vi "MGCC_FntStaMach_Visualization_OpalRT_demo_EvanEdit.vi"() -> ()   [LabVIEW 2016]
uses:
  Communication (Yiwei)/Global communication output.vi
panel:
  in  "test com":dbl[](array[numeric])
  in  "Matrix output":bool
  out "G14":bool
  out "G1":bool
  out "G6":bool
  out "L10":dbl
  in  "Tab Control 4":enum32{"Page 1"}(tab)
  out "PV Forecast":dbl[](graph)
  in  "Tab Control 3":enum32{"Page 1"}(tab)
  out "Sources Power":T1(graph)
  in  "Tab Control 2":enum32{"Page 1"}(tab)
  out "Frequency":T2(graph)
  in  "Irradiance":string(combo)="Manually Control"
  in  "island cmd 2":bool
  out "L11":dbl format="%#_4f"
  out "L9":dbl format="%#_4f"
  out "L7":dbl format="%#_4f"
  out "L8":dbl format="%#_4f"
  out "L4":dbl format="%#_4f"
  out "L3":dbl format="%#.1f"
  out "L2":dbl format="%#_4f"
  out "L5":dbl format="%#_4f"
  out "Total Load":dbl format="%#.1f"
  out "Max PV":dbl format="%#.1f"
  out "Resynchronization":bool
  out "Angle Diff.\n01-02":dbl format="%#.1f"
  out "Angle Diff.\n04-05":dbl format="%#.1f"
  out "Angle Diff.\n03-04":dbl format="%#.1f"
  out "Angle Diff.\n03-07":dbl format="%#.1f"
  out "Angle Diff.\n07-09":dbl format="%#.1f"
  out "Angle Diff.\n10-11":dbl format="%#.1f"
  out "L3":bool
  out "L2":bool
  out "2":cluster{dbl[], dbl[]}(graph)
  out "5":cluster{dbl[], dbl[]}(graph)
  out "4":cluster{dbl[], dbl[]}(graph)
  out "8":cluster{dbl[], dbl[]}(graph)
  out "9":cluster{dbl[], dbl[]}(graph)
  out "11":cluster{dbl[], dbl[]}(graph)
  in  "Stop":bool
  in  "RESET":bool
  out "3":cluster{dbl[], dbl[]}(graph)
  out "7":cluster{dbl[], dbl[]}(graph)
  out "10":cluster{dbl[], dbl[]}(graph)
  out "13":cluster{dbl[], dbl[]}(graph)
  out "14":cluster{dbl[], dbl[]}(graph)
  out "6":cluster{dbl[], dbl[]}(graph)
  out "1":cluster{dbl[], dbl[]}(graph)
  in  "Tab Control":T3(tab)
  out "Node Voltage":dbl(graph)
  out "Node Voltage":dbl(graph)
  out "Node Voltage":dbl(graph)
  out "Node Voltage":dbl(graph)
  out "Node Voltage":dbl(graph)
  out "Node Voltage":dbl(graph)
  out "Node Voltage":dbl(graph)
  out "Node Voltage":dbl(graph)
  out "Node Voltage":dbl(graph)
  out "Reactive power control":bool
  out "Active power control":bool
  out "Communication":bool
  out "Reactive power control":bool
  out "Active power control":bool
  out "Resynchronization":bool
  out "Communication":bool
  in  "Island 3":bool
  in  "Island 2":bool
  in  "Island":bool
  in  "Ready for STD":bool
  in  "Recon cmd":bool
  in  "BKS cmd":bool
  in  "island cmd":bool
  out "Angle Diff.\n11-14":dbl format="%#.1f"
  out "Angle Diff.\n09-10":dbl format="%#.1f"
  out "Angle Diff.\n04-06":dbl format="%#.1f"
  out "Angle Diff.\n 02-03":dbl format="%#.1f"
  out "BESS LC":bool
  out "PV LC":bool
  out "Topology Identification":bool
  out "PV Forecasting":bool
  out "Load Forecasting":bool
  out "PQ Balance":bool
  out "Black Start":bool
  out "Data Logging":bool
  out "Communication":bool
  out "State Estimation":bool
  out "Energy Mgmt.":bool
  out "SOC Tank":dbl(slide) scale=0.0..100.0
  out "S1114":bool
  out "S1011":bool
  out "S1012":bool
  out "S1013":bool
  out "S0910":bool
  out "S0708":bool
  out "S0709":bool
  out "S0307":bool
  out "S0304":bool
  out "S0406":bool
  out "S0405":bool
  out "S0203":bool
  out "S0102":bool
  out "W11":bool
  out "W8":bool
  out "L11":bool
  out "W12":bool
  out "L10":bool
  out "L7":bool
  out "L9":bool
  out "W7":bool
  out "L8":bool
  out "L4":bool
  out "L5":bool
  out "W6":bool
  out "W3":bool
  out "W2":bool
  out "Battery Output":dbl format="%#.1f"
  out "Battery SOC":dbl format="%#.1f"
  in  "PV-12":dbl(slide) scale=0.0..2.0
  out "PV Output":dbl format="%#.1f"
  out "W4":bool
  out "Current State":string
  out "W9":bool
  # "A Smart and Flexible Microgrid with a Low-cost Scalable Open-source Controller"
  # "Microgrid Central Controller"
  # "Battery Local Controller"
  # "%"
  # "G-6"
  # "kW"
  # "kW"
  # "kW"
  # "kW"
  # "kW"
  # "G-14"
  # "kW"
  # "kW"
  # "Deg"
  # "kW"
  # "Deg"
  # "Deg"
  # "kW"
  # "G-1"
  # "Deg"
  # "Deg"
  # "Deg"
  # "Deg"
  # "kW"
  # "Deg"
  # "kW"
  # "PV Local Controller"
  # "Deg"
  # "kW"
  # "kW"
  # "Deg"
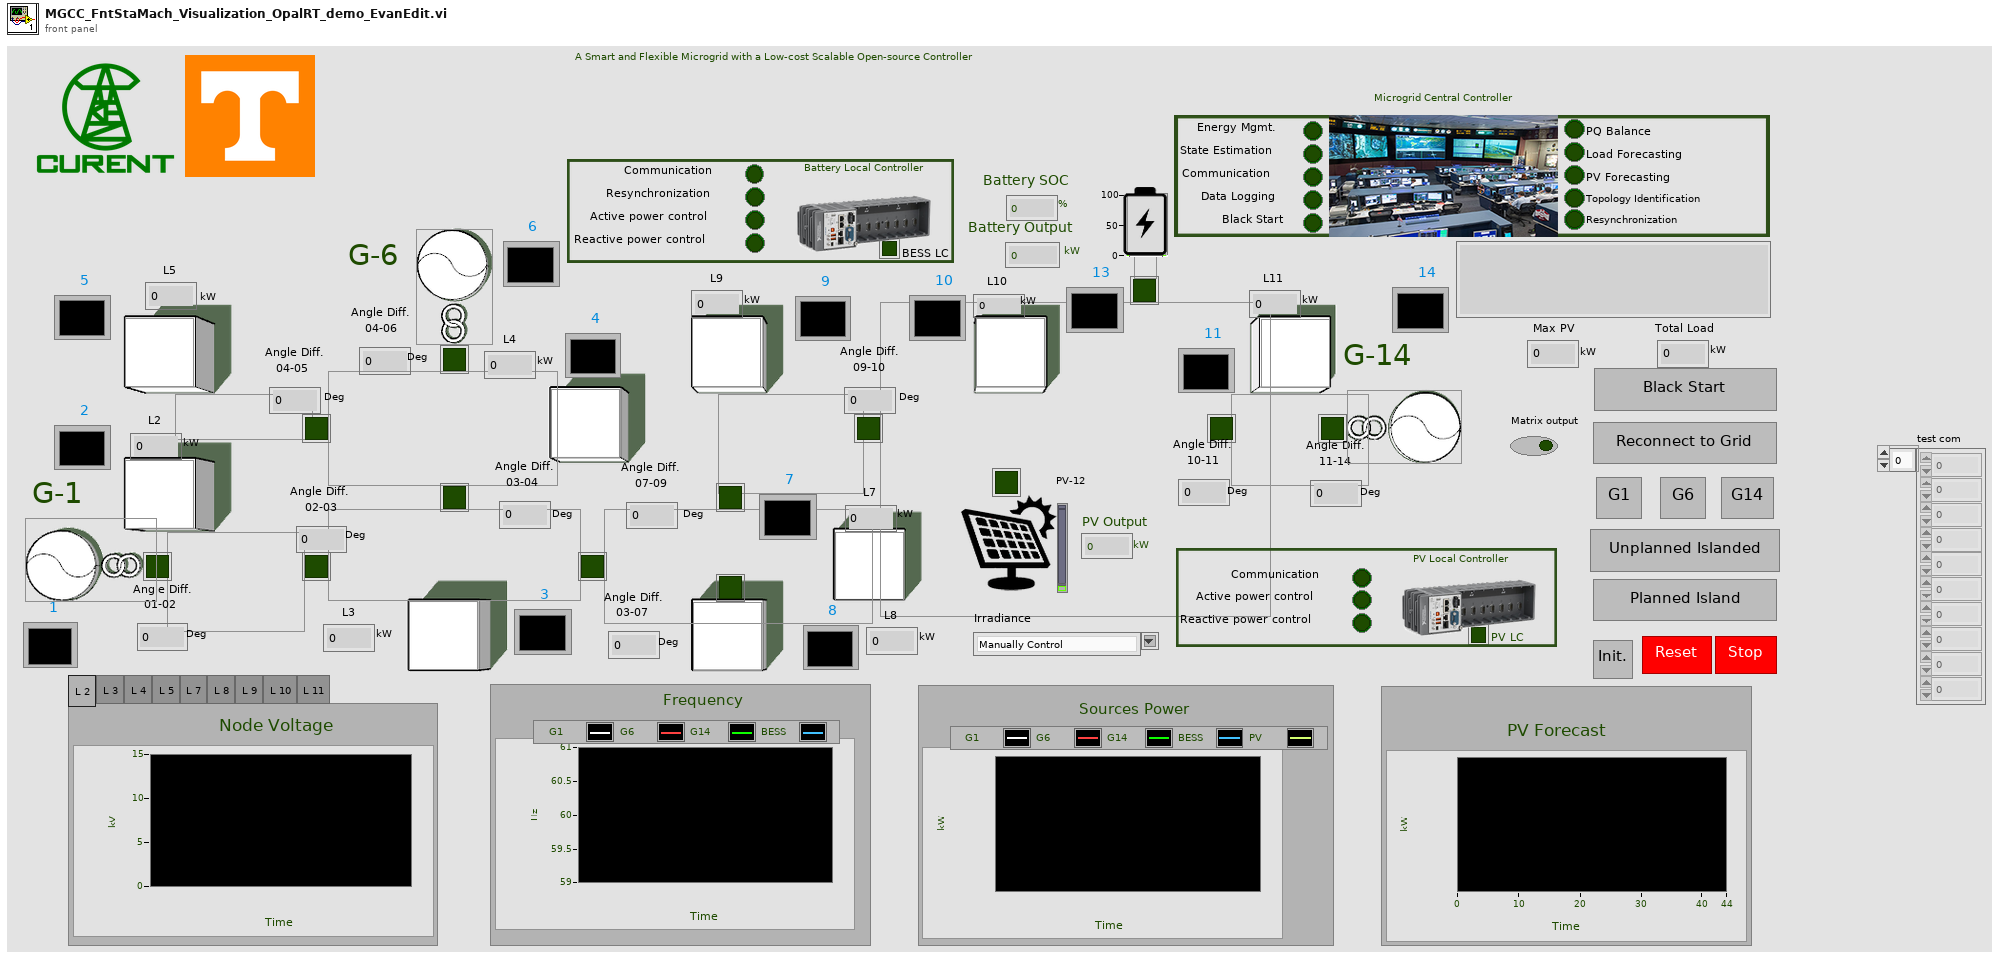
[diagram p1: front panel]
types:
  T1 = cluster{"Double":dbl, "Double":dbl, "Double":dbl, "Double":dbl, "Double":dbl}
  T2 = cluster{"Double":dbl, "Double":dbl, "Double":dbl, "Double":dbl}
  T3 = enum32{"L 2", "L 3", "L 4", "L 5", "L 7", "L 8", "L 9", "L 10", "L 11"}
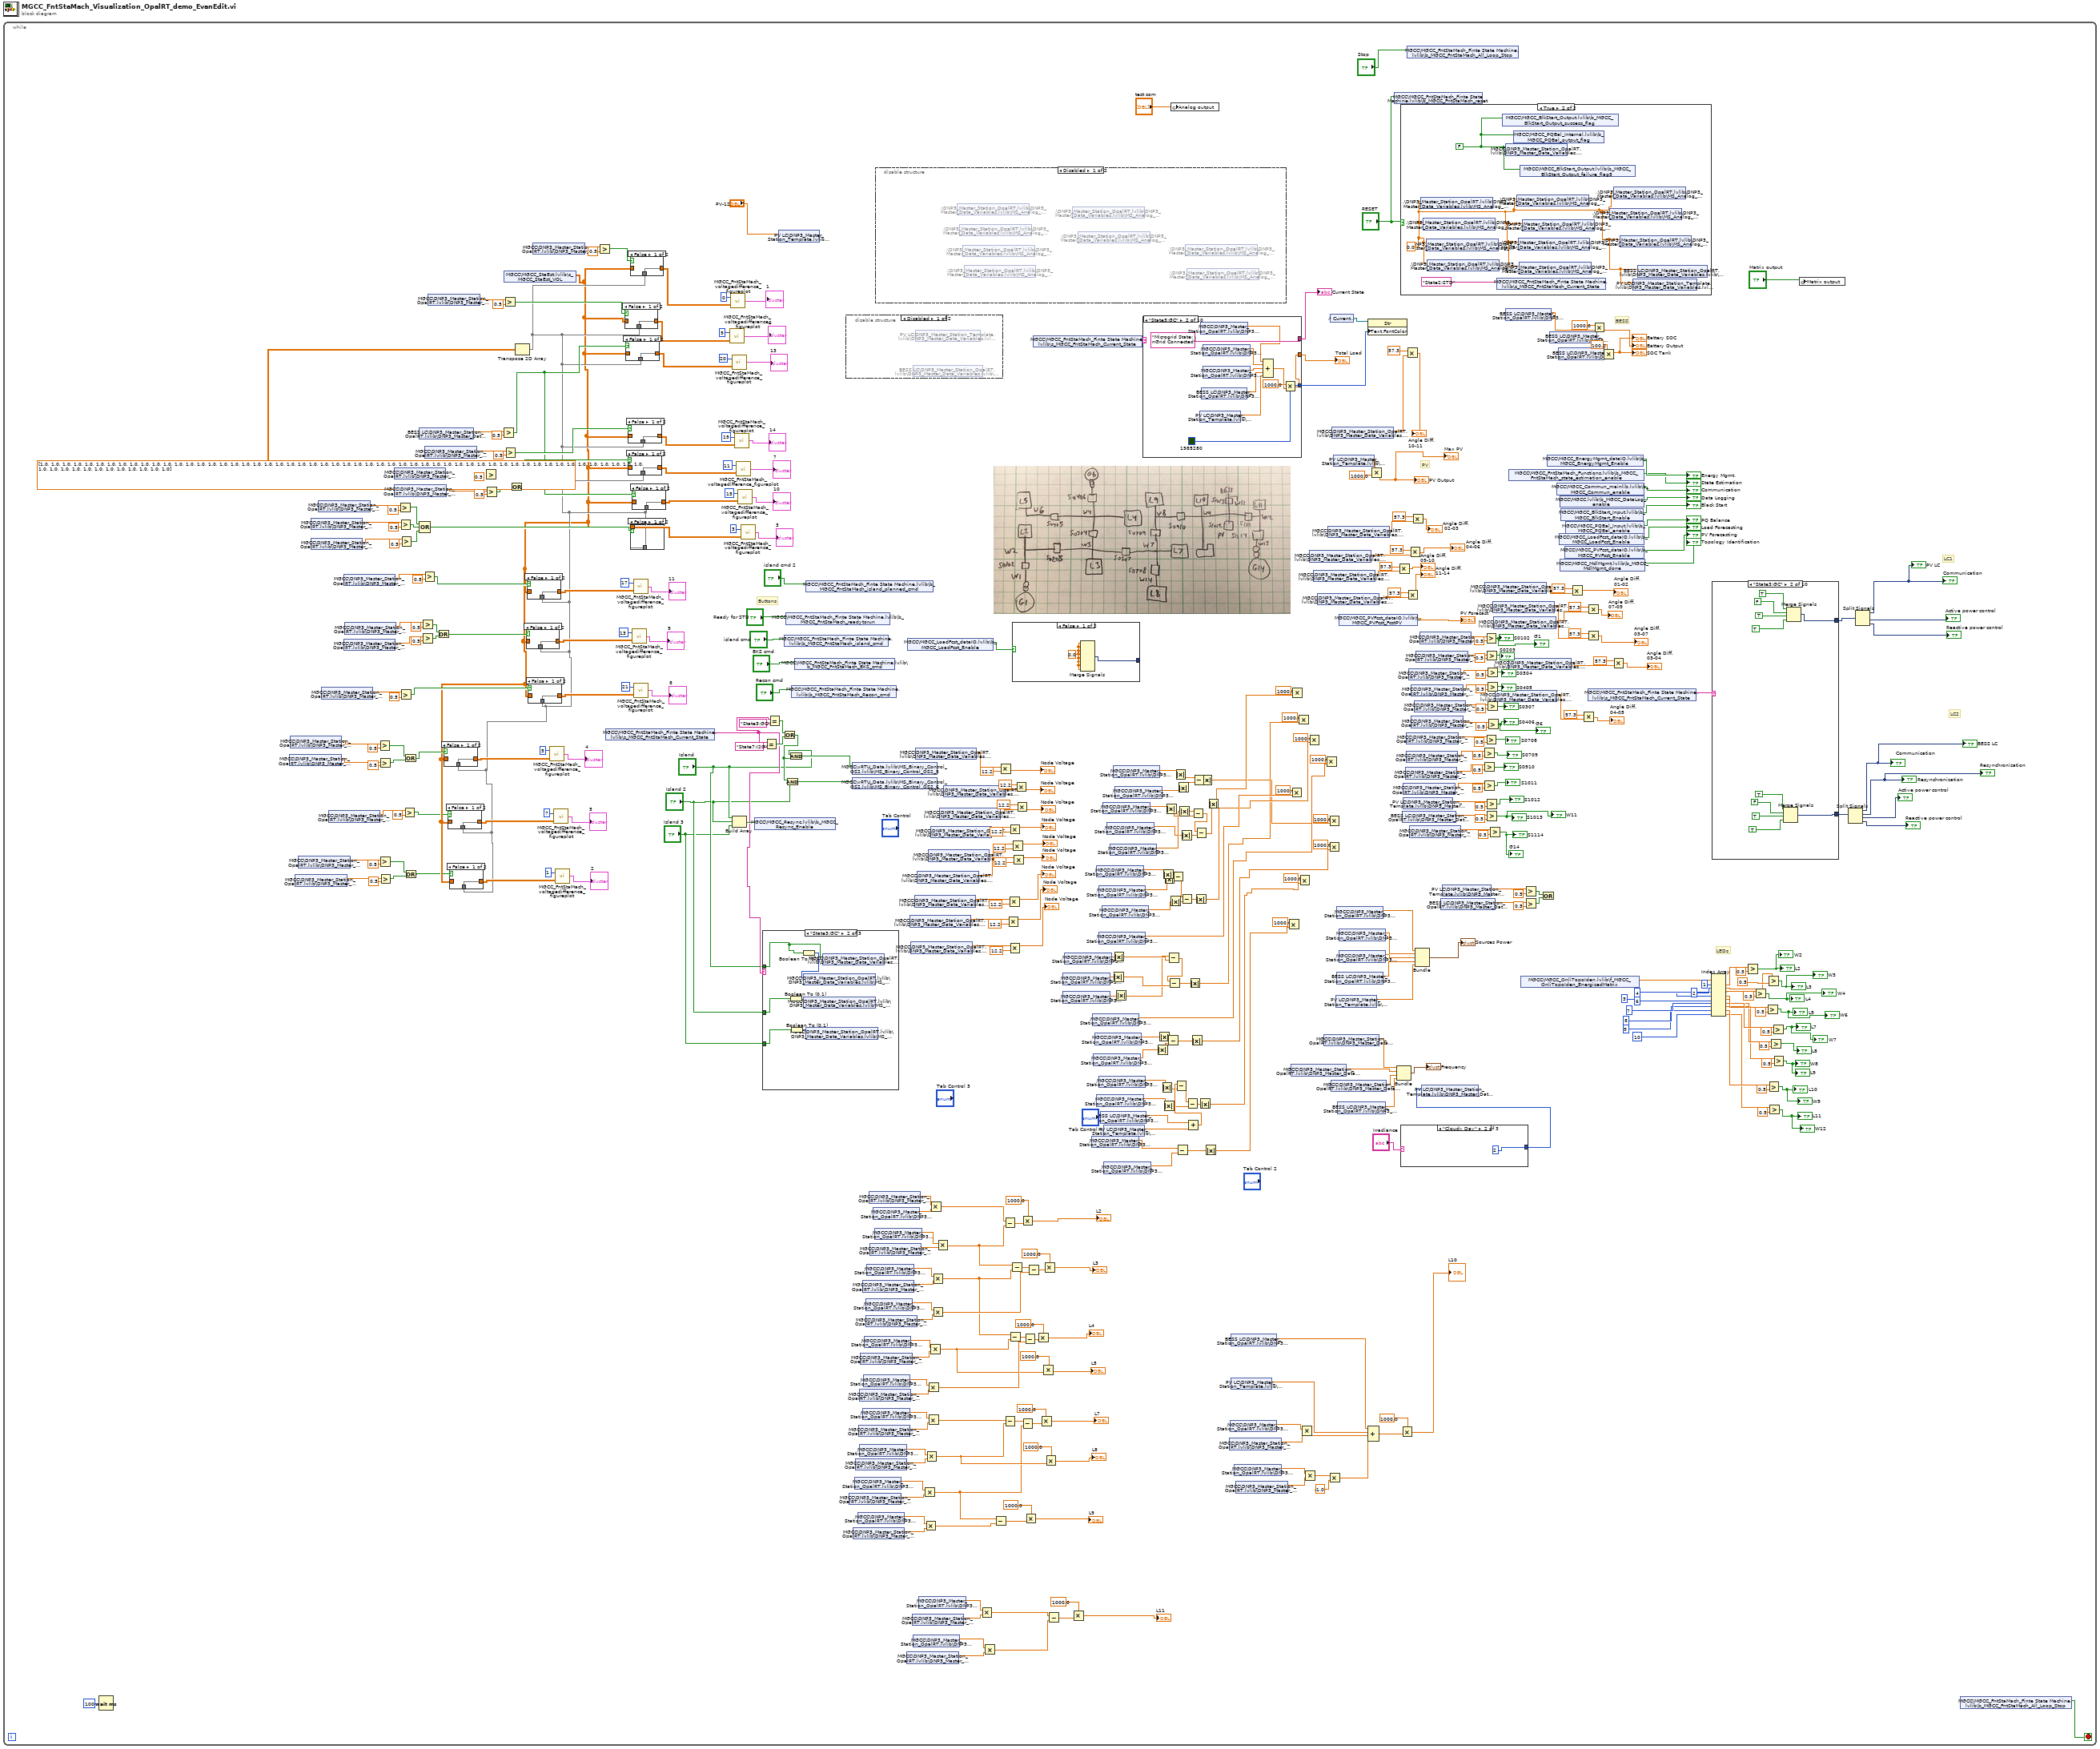
[diagram p0: block diagram]
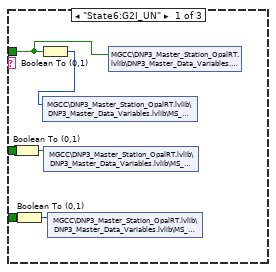
[diagram p2: hidden frame]
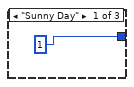
[diagram p4: hidden frame]
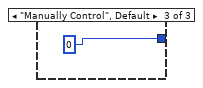
[diagram p5: hidden frame]
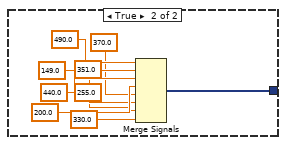
[diagram p6: hidden frame]
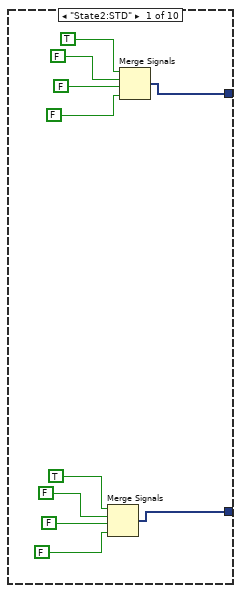
[diagram p7: hidden frame]
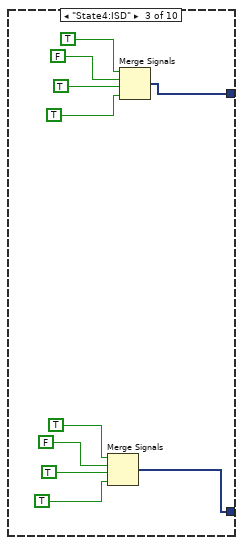
[diagram p8: hidden frame]
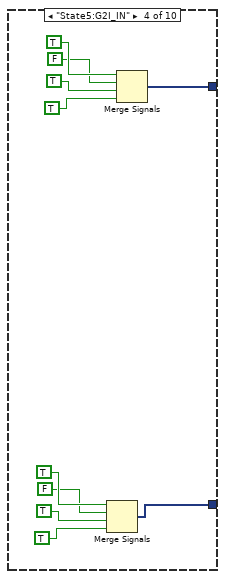
[diagram p9: hidden frame]
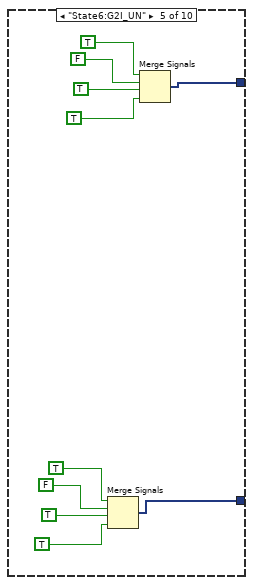
[diagram p10: hidden frame]
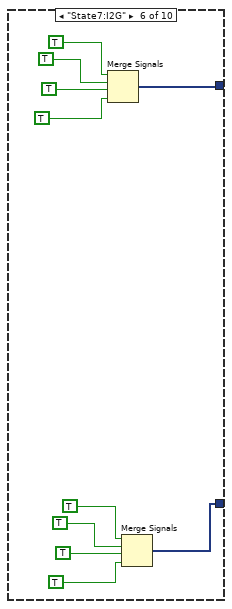
[diagram p11: hidden frame]
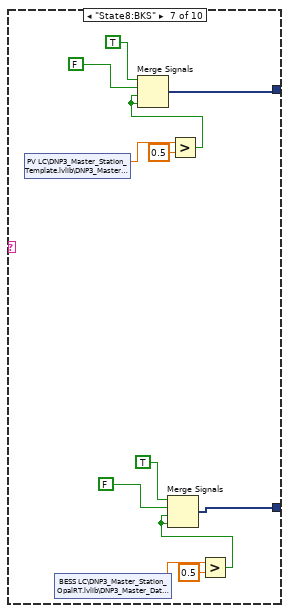
[diagram p12: hidden frame]
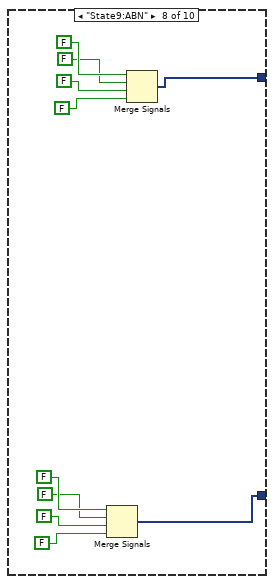
[diagram p13: hidden frame]
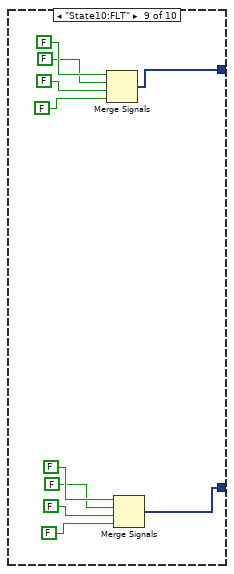
[diagram p14: hidden frame]
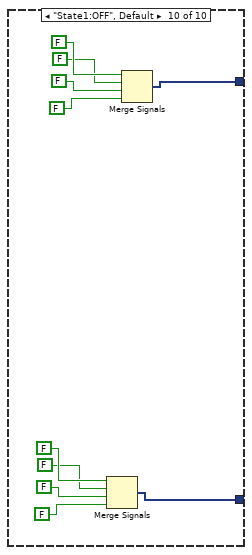
[diagram p15: hidden frame]
diagram:
  n1 = while {
    stop <- w2 stop-if-true
    # "LC1"
    # "LC2"
    # "PV"
    # "BESS"
    # "Buttons"
    # "LEDs"
    n2 = Wait (ms)(milliseconds to wait=u32 100) -> ()  [unwired: 1 out]
    n3 = shared-variable "MGCC\\DNP3_Master_Station_OpalRT.lvlib\\DNP3_Master_Data_Variables.lvlib\\MS_Analog_Status.lvlib\\S0406-status"() -> (w262:dbl)  [unwired: 1 in, 1 out]
    n4 = shared-variable "MGCC\\DNP3_Master_Station_OpalRT.lvlib\\DNP3_Master_Data_Variables.lvlib\\MS_Analog_Status.lvlib\\S0304-status"() -> (w263:dbl)  [unwired: 1 in, 1 out]
    n5 = shared-variable "MGCC\\DNP3_Master_Station_OpalRT.lvlib\\DNP3_Master_Data_Variables.lvlib\\MS_Analog_Status.lvlib\\S0203-status"() -> (w246:dbl)  [unwired: 1 in, 1 out]
    n6 = shared-variable "MGCC\\DNP3_Master_Station_OpalRT.lvlib\\DNP3_Master_Data_Variables.lvlib\\MS_Analog_Status.lvlib\\S0102-status"() -> (w247:dbl)  [unwired: 1 in, 1 out]
    n7 = shared-variable "MGCC\\DNP3_Master_Station_OpalRT.lvlib\\DNP3_Master_Data_Variables.lvlib\\MS_Analog_Status.lvlib\\S0307-status"() -> (w302:dbl)  [unwired: 1 in, 1 out]
    n8 = shared-variable "MGCC\\DNP3_Master_Station_OpalRT.lvlib\\DNP3_Master_Data_Variables.lvlib\\MS_Analog_Status.lvlib\\S0304-status"() -> (w303:dbl)  [unwired: 1 in, 1 out]
    n9 = shared-variable "MGCC\\DNP3_Master_Station_OpalRT.lvlib\\DNP3_Master_Data_Variables.lvlib\\MS_Analog_Status.lvlib\\S0203-status"() -> (w304:dbl)  [unwired: 1 in, 1 out]
    n10 = shared-variable "MGCC\\DNP3_Master_Station_OpalRT.lvlib\\DNP3_Master_Data_Variables.lvlib\\MS_Analog_Status.lvlib\\S0708-status"() -> (w269:dbl)  [unwired: 1 in, 1 out]
    n11 = shared-variable "MGCC\\DNP3_Master_Station_OpalRT.lvlib\\DNP3_Master_Data_Variables.lvlib\\MS_Analog_Status.lvlib\\S0405-status"() -> (w251:dbl)  [unwired: 1 in, 1 out]
    n12 = shared-variable "MGCC\\DNP3_Master_Station_OpalRT.lvlib\\DNP3_Master_Data_Variables.lvlib\\MS_Analog_Status.lvlib\\S1011-status"() -> (w288:dbl)  [unwired: 1 in, 1 out]
    n13 = shared-variable "MGCC\\DNP3_Master_Station_OpalRT.lvlib\\DNP3_Master_Data_Variables.lvlib\\MS_Analog_Status.lvlib\\S0910-status"() -> (w280:dbl)  [unwired: 1 in, 1 out]
    n14 = shared-variable "MGCC\\DNP3_Master_Station_OpalRT.lvlib\\DNP3_Master_Data_Variables.lvlib\\MS_Analog_Status.lvlib\\S0709-status"() -> (w281:dbl)  [unwired: 1 in, 1 out]
    n15 = Greater?(x=w263, y=0.5) -> (0:w265:bool)
    n16 = Greater?(x=w262, y=0.5) -> (0:w264:bool)
    n17 = Greater?(x=w247, y=0.5) -> (0:w245:bool)
    n18 = Greater?(x=w246, y=0.5) -> (0:w244:bool)
    n19 = shared-variable "MGCC\\DNP3_Master_Station_OpalRT.lvlib\\DNP3_Master_Data_Variables.lvlib\\MS_Analog_Status.lvlib\\S0307-status"() -> (w314:dbl)  [unwired: 1 in, 1 out]
    n20 = shared-variable "MGCC\\DNP3_Master_Station_OpalRT.lvlib\\DNP3_Master_Data_Variables.lvlib\\MS_Analog_Status.lvlib\\S0709-status"() -> (w313:dbl)  [unwired: 1 in, 1 out]
    n21 = Greater?(x=w304, y=0.5) -> (0:w301:bool)
    n22 = Greater?(x=w303, y=0.5) -> (0:w300:bool)
    n23 = Greater?(x=w269, y=0.5) -> (0:w268:bool)
    n24 = Greater?(x=w302, y=0.5) -> (0:w299:bool)
    n25 = Greater?(x=w251, y=0.5) -> (0:w250:bool)
    n26 = Or(x=w265, y=w264) -> (x .or. y?=w261:bool)
    n27 = Or(x=w245, y=w244) -> (x .or. y?=w243:bool)
    n28 = shared-variable "BESS LC\\DNP3_Master_Station_OpalRT.lvlib\\DNP3_Master_Data_Variables.lvlib\\MS_Analog_Status.lvlib\\BESS-STATUS"() -> (w326:dbl)  [unwired: 1 in, 1 out]
    n29 = Compound Arithmetic op=OR(w301, w300, w299) -> (w298:bool)
    n30 = Greater?(x=w281, y=0.5) -> (0:w279:bool)
    n31 = Greater?(x=w280, y=0.5) -> (0:w278:bool)
    n32 = Greater?(x=w288, y=0.5) -> (0:w287:bool)
    n33 = shared-variable "MGCC\\DNP3_Master_Station_OpalRT.lvlib\\DNP3_Master_Data_Variables.lvlib\\MS_Analog_Status.lvlib\\S1114-status"() -> (w320:dbl)  [unwired: 1 in, 1 out]
    n34 = shared-variable "MGCC\\DNP3_Master_Station_OpalRT.lvlib\\DNP3_Master_Data_Variables.lvlib\\MS_Analog_Status.lvlib\\S0406-status"() -> (w329:dbl)  [unwired: 1 in, 1 out]
    n35 = Or(x=w279, y=w278) -> (x .or. y?=w277:bool)
    n36 = Greater?(x=w314, y=0.5) -> (0:w316:bool)
    n37 = Greater?(x=w313, y=0.5) -> (0:w315:bool)
    n38 = Greater?(x=w326, y=0.5) -> (0:w311:bool)
    n39 = Greater?(x=w329, y=0.5) -> (0:w328:bool)
    n40 = Greater?(x=w320, y=0.5) -> (0:w319:bool)
    n41 = shared-variable "MGCC\\MGCC_StaEst.lvlib\\c_MGCC_StaEst_VOL"() -> (w253:cdb[][])  [unwired: 1 in, 1 out]
    n42 = Or(x=w316, y=w315) -> (x .or. y?=w312:bool)
    n43 = Transpose 2D Array(2D array=dbl[][] [[1.0, 1.0, 1.0, 1.0, 1.0, 1.0, 1.0, 1.0, 1.0, 1.0, 1.0, 1.0, 1.0, 1.0, 1.0, 1.0, 1.0, 1.0, 1.0, 1.0, 1.0, 1.0], [1.0, 1.0, 1.0, 1.0, 1.0, 1.0, 1.0, 1.0, 1.0, 1.0, 1.0, 1.0, 1.0, 1.0, 1.0, 1.0, 1.0, 1.0, 1.0, 1.0, 1.0, 1.0], [1.0, 1.0, 1.0, 1.0, 1.0, 1.0, 1.0, 1.0, 1.0, 1.0, 1.0, 1.0, 1.0, 1.0, 1.0, 1.0, 1.0, 1.0, 1.0, 1.0, 1.0, 1.0]] ("lower limit")) -> (transposed array=w254:dbl[][])
    n44 = case shown="False" w261 {
      tunnel: w253 -> [_ w584]
      tunnel: [w583 w584] -> w271
      tunnel: w254 -> [w583 _]
      frame False {
      }
      frame True {
      }
    }
    n45 = case shown="False" w250 {
      tunnel: w253 -> [_ w582]
      tunnel: [w581 w582] -> w258
      tunnel: w254 -> [w581 _]
      frame False {
      }
      frame True {
      }
    }
    n46 = case shown="False" w243 {
      tunnel: w253 -> [_ w580]
      tunnel: [w579 w580] -> w255
      tunnel: w254 -> [w579 _]
      frame False {
      }
      frame True {
      }
    }
    n47 = case shown="False" w277 {
      tunnel: w253 -> [_ w588]
      tunnel: [w587 w588] -> w284
      tunnel: w254 -> [w587 _]
      frame False {
      }
      frame True {
      }
    }
    n48 = case shown="False" w287 {
      tunnel: w253 -> [_ w590]
      tunnel: [w589 w590] -> w290
      tunnel: w254 -> [w589 _]
      frame False {
      }
      frame True {
      }
    }
    n49 = case shown="False" w268 {
      tunnel: w253 -> [_ w586]
      tunnel: [w585 w586] -> w274
      tunnel: w254 -> [w585 _]
      frame False {
      }
      frame True {
      }
    }
    n50 = shared-variable "MGCC\\DNP3_Master_Station_OpalRT.lvlib\\DNP3_Master_Data_Variables.lvlib\\MS_Analog_Status.lvlib\\S0102-status"() -> (w333:dbl)  [unwired: 1 in, 1 out]
    n51 = call "MGCC_FntStaMach_voltagedifference_figureplot.vi"("array"=w271, "index (row)"=5) -> ("output cluster"=→"4":cluster{dbl[], dbl[]})
    n52 = call "MGCC_FntStaMach_voltagedifference_figureplot.vi"("array"=w258, "index (row)"=7) -> ("output cluster"=→"5":cluster{dbl[], dbl[]})
    n53 = call "MGCC_FntStaMach_voltagedifference_figureplot.vi"("array"=w255, "index (row)"=1) -> ("output cluster"=→"2":cluster{dbl[], dbl[]})
    n54 = Greater?(x=w333, y=0.5) -> (0:w332:bool)
    n55 = shared-variable "MGCC\\MGCC_FntStaMach_Finte State Machine.lvlib\\s_MGCC_FntStaMach_Current_State"() -> (w83:string)  [unwired: 1 in, 1 out]
    n56 = case shown="False" w328 {
      tunnel: w253 -> [_ w666]
      tunnel: [w665 w666] -> w331
      tunnel: w254 -> [w665 _]
      frame False {
      }
      frame True {
      }
    }
    n57 = case shown="False" w311 {
      tunnel: w253 -> [_ w664]
      tunnel: [w663 w664] -> w325
      tunnel: w254 -> [w663 _]
      frame False {
      }
      frame True {
      }
    }
    n58 = case shown="False" w319 {
      tunnel: w253 -> [_ w662]
      tunnel: [w661 w662] -> w324
      tunnel: w254 -> [w661 _]
      frame False {
      }
      frame True {
      }
    }
    n59 = case shown="False" w312 {
      tunnel: w253 -> [_ w660]
      tunnel: [w659 w660] -> w323
      tunnel: w254 -> [w659 _]
      frame False {
      }
      frame True {
      }
    }
    n60 = case shown="False" w332 {
      tunnel: w253 -> [_ w668]
      tunnel: [w667 w668] -> w335
      tunnel: w254 -> [w667 _]
      frame False {
      }
      frame True {
      }
    }
    n61 = case shown="False" w298 {
      tunnel: w253 -> [_ w656]
      tunnel: [w655 w656] -> w308
      tunnel: w254 -> [w655 _]
      frame False {
      }
      frame True {
      }
    }
    n62 = case shown="False" w311 {
      tunnel: w253 -> [_ w658]
      tunnel: [w657 w658] -> w322
      tunnel: w254 -> [w657 _]
      frame False {
      }
      frame True {
      }
    }
    n63 = call "MGCC_FntStaMach_voltagedifference_figureplot.vi"("array"=w284, "index (row)"=13) -> ("output cluster"=→"9":cluster{dbl[], dbl[]})
    n64 = call "MGCC_FntStaMach_voltagedifference_figureplot.vi"("array"=w290, "index (row)"=17) -> ("output cluster"=→"11":cluster{dbl[], dbl[]})
    n65 = call "MGCC_FntStaMach_voltagedifference_figureplot.vi"("array"=w274, "index (row)"=21) -> ("output cluster"=→"8":cluster{dbl[], dbl[]})
    n66 = call "MGCC_FntStaMach_voltagedifference_figureplot.vi"("array"=w331, "index (row)"=9) -> ("output cluster"=→"6":cluster{dbl[], dbl[]})
    n67 = call "MGCC_FntStaMach_voltagedifference_figureplot.vi"("array"=w335, "index (row)"=0) -> ("output cluster"=→"1":cluster{dbl[], dbl[]})
    n68 = call "MGCC_FntStaMach_voltagedifference_figureplot.vi"("array"=w325, "index (row)"=20) -> ("output cluster"=→"13":cluster{dbl[], dbl[]})
    n69 = Build Array("Island", "Island 2", "Island 3") -> (w235:bool[])
    n70 = call "MGCC_FntStaMach_voltagedifference_figureplot.vi"("array"=w324, "index (row)"=19) -> ("output cluster"=→"14":cluster{dbl[], dbl[]})
    n71 = call "MGCC_FntStaMach_voltagedifference_figureplot.vi"("array"=w323, "index (row)"=11) -> ("output cluster"=→"7":cluster{dbl[], dbl[]})
    n72 = call "MGCC_FntStaMach_voltagedifference_figureplot.vi"("array"=w322, "index (row)"=15) -> ("output cluster"=→"10":cluster{dbl[], dbl[]})
    n73 = call "MGCC_FntStaMach_voltagedifference_figureplot.vi"("array"=w308, "index (row)"=3) -> ("output cluster"=→"3":cluster{dbl[], dbl[]})
    n74 = shared-variable "MGCC\\MGCC_Resync.lvlib\\b_MGCC_Resync_Enable"(w235) -> ()  [unwired: 1 in, 1 out]
    n75 = case shown="\"State3:GC\"" w83 {
      tunnel: "Island" -> [w451 w457 _]
      tunnel: "Island 2" -> [w455 w459 _]
      tunnel: "Island 3" -> [w453 w458 _]
      frame "State6:G2I_UN" {
        n76 = Boolean To (0,1)(Boolean=w455) -> (0, 1=w454:i16)
        n77 = Boolean To (0,1)(Boolean=w453) -> (0, 1=w452:i16)
        n78 = Boolean To (0,1)(Boolean=w451) -> (0, 1=w456:i16)
        n79 = shared-variable "MGCC\\DNP3_Master_Station_OpalRT.lvlib\\DNP3_Master_Data_Variables.lvlib\\MS_Analog_Control.lvlib\\S0102-STATUS-CTRL"(w456) -> ()  [unwired: 1 in, 1 out]
        n80 = shared-variable "MGCC\\DNP3_Master_Station_OpalRT.lvlib\\DNP3_Master_Data_Variables.lvlib\\MS_Analog_Control.lvlib\\S0406-STATUS-CTRL"(w454) -> ()  [unwired: 1 in, 1 out]
        n81 = shared-variable "MGCC\\DNP3_Master_Station_OpalRT.lvlib\\DNP3_Master_Data_Variables.lvlib\\MS_Analog_Control.lvlib\\S1114-STATUS-CTRL"(w452) -> ()  [unwired: 1 in, 1 out]
        n82 = shared-variable "MGCC\\DNP3_Master_Station_OpalRT.lvlib\\DNP3_Master_Data_Variables.lvlib\\MS_Binary_Control.lvlib\\S0102-status-ctrl"(w451) -> ()  [unwired: 1 in, 1 out]
      }
      frame "State3:GC" {
        n83 = Boolean To (0,1)(Boolean=w459) -> (0, 1=w461:i16)
        n84 = Boolean To (0,1)(Boolean=w458) -> (0, 1=w460:i16)
        n85 = Boolean To (0,1)(Boolean=w457) -> (0, 1=w462:i16)
        n86 = shared-variable "MGCC\\DNP3_Master_Station_OpalRT.lvlib\\DNP3_Master_Data_Variables.lvlib\\MS_Analog_Control.lvlib\\S0102-STATUS-CTRL"(w462) -> ()  [unwired: 1 in, 1 out]
        n87 = shared-variable "MGCC\\DNP3_Master_Station_OpalRT.lvlib\\DNP3_Master_Data_Variables.lvlib\\MS_Analog_Control.lvlib\\S0406-STATUS-CTRL"(w461) -> ()  [unwired: 1 in, 1 out]
        n88 = shared-variable "MGCC\\DNP3_Master_Station_OpalRT.lvlib\\DNP3_Master_Data_Variables.lvlib\\MS_Analog_Control.lvlib\\S1114-STATUS-CTRL"(w460) -> ()  [unwired: 1 in, 1 out]
        n89 = shared-variable "MGCC\\DNP3_Master_Station_OpalRT.lvlib\\DNP3_Master_Data_Variables.lvlib\\MS_Binary_Control.lvlib\\S0102-status-ctrl"(w457) -> ()  [unwired: 1 in, 1 out]
      }
      frame "False", Default {
      }
    }
    n90 = Equal?(x=w83, y="State7:I2G") -> (x = y?=w434:bool)
    n91 = Equal?(x=w83, y="State3:GC") -> (x = y?=w433:bool)
    n92 = shared-variable "PV LC\\DNP3_Master_Station_Template.lvlib\\DNP3_Master_Data_Variables.lvlib\\MS_Analog_Control.lvlib\\PV-APC"("PV-12") -> ()  [unwired: 1 in, 1 out]
    n93 = Or(x=w433, y=w434) -> (x .or. y?=w432:bool)
    n94 = shared-variable "MGCC\\MGCC_FntStaMach_Finte State Machine.lvlib\\b_MGCC_FntStaMach_island_cmd"("island cmd") -> ()  [unwired: 1 in, 1 out]
    n95 = And(x=w432, y="Island 2") -> (x .and. y?=w430:bool)
    n96 = shared-variable "MGCC\\MGCC_FntStaMach_Finte State Machine.lvlib\\b_MGCC_FntStaMach_readytorun"("Ready for STD") -> ()  [unwired: 1 in, 1 out]
    n97 = And(x="Island", y=w432) -> (x .and. y?=w431:bool)
    n98 = shared-variable "MGCC\\MGCC_FntStaMach_Finte State Machine.lvlib\\b_MGCC_FntStaMach_Recon_cmd"("Recon cmd") -> ()  [unwired: 1 in, 1 out]
    n99 = shared-variable "MGCC\\MGCC_FntStaMach_Finte State Machine.lvlib\\b_MGCC_FntStaMach_BKS_cmd"("BKS cmd") -> ()  [unwired: 1 in, 1 out]
    n100 = shared-variable "MGCC\\MGCC_FntStaMach_Finte State Machine.lvlib\\b_MGCC_FntStaMach_island_planned_cmd"("island cmd 2") -> ()  [unwired: 1 in, 1 out]
    n101 = disable-structure shown="Disabled" {
      frame Disabled {
        n102 = shared-variable "BESS LC\\DNP3_Master_Station_OpalRT.lvlib\\DNP3_Master_Data_Variables.lvlib\\MS_Analog_Control.lvlib\\BESS-STATUS-CTRL"() -> (w654:dbl)  [unwired: 1 in, 1 out]
        n103 = shared-variable "PV LC\\DNP3_Master_Station_Template.lvlib\\DNP3_Master_Data_Variables.lvlib\\MS_Analog_Control.lvlib\\PV-STATUS-CTRL"() -> (w653:dbl)  [unwired: 1 in, 1 out]
      }
      frame Enabled {
      }
    }
    n104 = shared-variable "MGCC\\DNP3_Master_Station_OpalRT.lvlib\\DNP3_Master_Data_Variables.lvlib\\MS_Analog_Status.lvlib\\S0709-status"() -> (w49:dbl)  [unwired: 1 in, 1 out]
    n105 = shared-variable "MGCC\\vRTU_Data.lvlib\\MS_Binary_Control_OS2.lvlib\\MS_Binary_Control_OS2_5"(w431) -> ()  [unwired: 1 in, 1 out]
    n106 = shared-variable "MGCC\\vRTU_Data.lvlib\\MS_Binary_Control_OS2.lvlib\\MS_Binary_Control_OS2_6"(w430) -> ()  [unwired: 1 in, 1 out]
    n107 = shared-variable "MGCC\\DNP3_Master_Station_OpalRT.lvlib\\DNP3_Master_Data_Variables.lvlib\\MS_Analog_Status.lvlib\\S0910-status"() -> (w47:dbl)  [unwired: 1 in, 1 out]
    n108 = shared-variable "MGCC\\DNP3_Master_Station_OpalRT.lvlib\\DNP3_Master_Data_Variables.lvlib\\MS_Analog_Status.lvlib\\S0709-APF"() -> (w50:dbl)  [unwired: 1 in, 1 out]
    n109 = shared-variable "MGCC\\DNP3_Master_Station_OpalRT.lvlib\\DNP3_Master_Data_Variables.lvlib\\MS_Analog_Status.lvlib\\S0708-status"() -> (w51:dbl)  [unwired: 1 in, 1 out]
    n110 = shared-variable "MGCC\\DNP3_Master_Station_OpalRT.lvlib\\DNP3_Master_Data_Variables.lvlib\\MS_Analog_Status.lvlib\\S0910-APF"() -> (w48:dbl)  [unwired: 1 in, 1 out]
    n111 = shared-variable "MGCC\\DNP3_Master_Station_OpalRT.lvlib\\DNP3_Master_Data_Variables.lvlib\\MS_Analog_Status.lvlib\\S0307-status"() -> (w53:dbl)  [unwired: 1 in, 1 out]
    n112 = shared-variable "MGCC\\DNP3_Master_Station_OpalRT.lvlib\\DNP3_Master_Data_Variables.lvlib\\MS_Analog_Status.lvlib\\S0406-status"() -> (w55:dbl)  [unwired: 1 in, 1 out]
    n113 = shared-variable "MGCC\\DNP3_Master_Station_OpalRT.lvlib\\DNP3_Master_Data_Variables.lvlib\\MS_Analog_Status.lvlib\\S0708-APF"() -> (w52:dbl)  [unwired: 1 in, 1 out]
    n114 = shared-variable "MGCC\\DNP3_Master_Station_OpalRT.lvlib\\DNP3_Master_Data_Variables.lvlib\\MS_Analog_Status.lvlib\\S0405-status"() -> (w57:dbl)  [unwired: 1 in, 1 out]
    n115 = shared-variable "MGCC\\DNP3_Master_Station_OpalRT.lvlib\\DNP3_Master_Data_Variables.lvlib\\MS_Analog_Status.lvlib\\S0304-status"() -> (w61:dbl)  [unwired: 1 in, 1 out]
    n116 = shared-variable "MGCC\\DNP3_Master_Station_OpalRT.lvlib\\DNP3_Master_Data_Variables.lvlib\\MS_Analog_Status.lvlib\\S0307-APF"() -> (w54:dbl)  [unwired: 1 in, 1 out]
    n117 = shared-variable "MGCC\\DNP3_Master_Station_OpalRT.lvlib\\DNP3_Master_Data_Variables.lvlib\\MS_Analog_Status.lvlib\\S0406-APF"() -> (w56:dbl)  [unwired: 1 in, 1 out]
    n118 = shared-variable "MGCC\\DNP3_Master_Station_OpalRT.lvlib\\DNP3_Master_Data_Variables.lvlib\\MS_Analog_Status.lvlib\\S0405-APF"() -> (w58:dbl)  [unwired: 1 in, 1 out]
    n119 = shared-variable "MGCC\\DNP3_Master_Station_OpalRT.lvlib\\DNP3_Master_Data_Variables.lvlib\\MS_Analog_Status.lvlib\\S0307-APF"() -> (w60:dbl)  [unwired: 1 in, 1 out]
    n120 = shared-variable "MGCC\\DNP3_Master_Station_OpalRT.lvlib\\DNP3_Master_Data_Variables.lvlib\\MS_Analog_Status.lvlib\\S0307-status"() -> (w59:dbl)  [unwired: 1 in, 1 out]
    n121 = shared-variable "MGCC\\DNP3_Master_Station_OpalRT.lvlib\\DNP3_Master_Data_Variables.lvlib\\MS_Analog_Status.lvlib\\S0304-APF"() -> (w62:dbl)  [unwired: 1 in, 1 out]
    n122 = shared-variable "MGCC\\DNP3_Master_Station_OpalRT.lvlib\\DNP3_Master_Data_Variables.lvlib\\MS_Analog_Status.lvlib\\S0102-status"() -> (w66:dbl)  [unwired: 1 in, 1 out]
    n123 = shared-variable "MGCC\\DNP3_Master_Station_OpalRT.lvlib\\DNP3_Master_Data_Variables.lvlib\\MS_Analog_Status.lvlib\\S0203-status"() -> (w63:dbl)  [unwired: 1 in, 1 out]
    n124 = shared-variable "MGCC\\DNP3_Master_Station_OpalRT.lvlib\\DNP3_Master_Data_Variables.lvlib\\MS_Analog_Status.lvlib\\S0102-APF"() -> (w65:dbl)  [unwired: 1 in, 1 out]
    n125 = shared-variable "MGCC\\DNP3_Master_Station_OpalRT.lvlib\\DNP3_Master_Data_Variables.lvlib\\MS_Analog_Status.lvlib\\S0203-APF"() -> (w64:dbl)  [unwired: 1 in, 1 out]
    n126 = disable-structure shown="Disabled" {
      frame Disabled {
        n127 = shared-variable ".\\DNP3_Master_Station_OpalRT.lvlib\\DNP3_Master_Data_Variables.lvlib\\MS_Analog_Control.lvlib\\S0203-STATUS-CTRL"() -> (w652:dbl)  [unwired: 1 in, 1 out]
        n128 = shared-variable ".\\DNP3_Master_Station_OpalRT.lvlib\\DNP3_Master_Data_Variables.lvlib\\MS_Analog_Control.lvlib\\S0304-STATUS-CTRL"() -> (w651:dbl)  [unwired: 1 in, 1 out]
        n129 = shared-variable ".\\DNP3_Master_Station_OpalRT.lvlib\\DNP3_Master_Data_Variables.lvlib\\MS_Analog_Control.lvlib\\S0307-STATUS-CTRL"() -> (w650:dbl)  [unwired: 1 in, 1 out]
        n130 = shared-variable ".\\DNP3_Master_Station_OpalRT.lvlib\\DNP3_Master_Data_Variables.lvlib\\MS_Analog_Control.lvlib\\S0405-STATUS-CTRL"() -> (w649:dbl)  [unwired: 1 in, 1 out]
        n131 = shared-variable ".\\DNP3_Master_Station_OpalRT.lvlib\\DNP3_Master_Data_Variables.lvlib\\MS_Analog_Control.lvlib\\S0708-STATUS-CTRL"() -> (w648:dbl)  [unwired: 1 in, 1 out]
        n132 = shared-variable ".\\DNP3_Master_Station_OpalRT.lvlib\\DNP3_Master_Data_Variables.lvlib\\MS_Analog_Control.lvlib\\S0709-STATUS-CTRL"() -> (w647:dbl)  [unwired: 1 in, 1 out]
        n133 = shared-variable ".\\DNP3_Master_Station_OpalRT.lvlib\\DNP3_Master_Data_Variables.lvlib\\MS_Analog_Control.lvlib\\S0910-STATUS-CTRL"() -> (w646:dbl)  [unwired: 1 in, 1 out]
        n134 = shared-variable ".\\DNP3_Master_Station_OpalRT.lvlib\\DNP3_Master_Data_Variables.lvlib\\MS_Analog_Control.lvlib\\S1011-STATUS-CTRL"() -> (w645:dbl)  [unwired: 1 in, 1 out]
      }
      frame Enabled {
      }
    }
    n135 = shared-variable "MGCC\\DNP3_Master_Station_OpalRT.lvlib\\DNP3_Master_Data_Variables.lvlib\\MS_Analog_Status.lvlib\\S1114-status"() -> (w43:dbl)  [unwired: 1 in, 1 out]
    n136 = shared-variable "MGCC\\MGCC_LoadFcst_dataIO.lvlib\\b_MGCC_LoadFcst_Enable"() -> (w116:bool)  [unwired: 1 in, 1 out]
    n137 = shared-variable "MGCC\\DNP3_Master_Station_OpalRT.lvlib\\DNP3_Master_Data_Variables.lvlib\\MS_Analog_Status.lvlib\\S0910-MAG-A-R"() -> (w422:dbl)  [unwired: 1 in, 1 out]
    n138 = shared-variable "MGCC\\DNP3_Master_Station_OpalRT.lvlib\\DNP3_Master_Data_Variables.lvlib\\MS_Analog_Status.lvlib\\S1011-MAG-A-R"() -> (w421:dbl)  [unwired: 1 in, 1 out]
    n139 = shared-variable "MGCC\\DNP3_Master_Station_OpalRT.lvlib\\DNP3_Master_Data_Variables.lvlib\\MS_Analog_Status.lvlib\\S1011-status"() -> (w45:dbl)  [unwired: 1 in, 1 out]
    n140 = shared-variable "MGCC\\DNP3_Master_Station_OpalRT.lvlib\\DNP3_Master_Data_Variables.lvlib\\MS_Analog_Status.lvlib\\S1114-APF"() -> (w44:dbl)  [unwired: 1 in, 1 out]
    n141 = shared-variable "MGCC\\DNP3_Master_Station_OpalRT.lvlib\\DNP3_Master_Data_Variables.lvlib\\MS_Analog_Status.lvlib\\S0709-MAG-A-R"() -> (w423:dbl)  [unwired: 1 in, 1 out]
    n142 = shared-variable "MGCC\\DNP3_Master_Station_OpalRT.lvlib\\DNP3_Master_Data_Variables.lvlib\\MS_Analog_Status.lvlib\\S0102-MAG-A-R"() -> (w429:dbl)  [unwired: 1 in, 1 out]
    n143 = shared-variable "MGCC\\DNP3_Master_Station_OpalRT.lvlib\\DNP3_Master_Data_Variables.lvlib\\MS_Analog_Status.lvlib\\S0708-MAG-A-R"() -> (w424:dbl)  [unwired: 1 in, 1 out]
    n144 = shared-variable "MGCC\\DNP3_Master_Station_OpalRT.lvlib\\DNP3_Master_Data_Variables.lvlib\\MS_Analog_Status.lvlib\\S1011-APF"() -> (w46:dbl)  [unwired: 1 in, 1 out]
    n145 = Multiply(x=w50, y=w49) -> (x*y=w21:dbl)
    n146 = Multiply(x=w48, y=w47) -> (x*y=w20:dbl)
    n147 = Multiply(x=w52, y=w51) -> (x*y=w22:dbl)
    n148 = Multiply(x=w56, y=w55) -> (x*y=w32:dbl)
    n149 = Multiply(x=w54, y=w53) -> (x*y=w27:dbl)
    n150 = shared-variable "MGCC\\DNP3_Master_Station_OpalRT.lvlib\\DNP3_Master_Data_Variables.lvlib\\MS_Analog_Status.lvlib\\S0307-MAG-A-R"() -> (w425:dbl)  [unwired: 1 in, 1 out]
    n151 = Multiply(x=w58, y=w57) -> (x*y=w28:dbl)
    n152 = Multiply(x=w66, y=w65) -> (x*y=w42:dbl)
    n153 = shared-variable "MGCC\\DNP3_Master_Station_OpalRT.lvlib\\DNP3_Master_Data_Variables.lvlib\\MS_Analog_Status.lvlib\\S0405-MAG-A-R"() -> (w426:dbl)  [unwired: 1 in, 1 out]
    n154 = Multiply(x=w62, y=w61) -> (x*y=w34:dbl)
    n155 = Multiply(x=w60, y=w59) -> (x*y=w37:dbl)
    n156 = Multiply(x=w64, y=w63) -> (x*y=w39:dbl)
    n157 = shared-variable "MGCC\\DNP3_Master_Station_OpalRT.lvlib\\DNP3_Master_Data_Variables.lvlib\\MS_Analog_Status.lvlib\\S0304-MAG-A-R"() -> (w427:dbl)  [unwired: 1 in, 1 out]
    n158 = shared-variable "MGCC\\DNP3_Master_Station_OpalRT.lvlib\\DNP3_Master_Data_Variables.lvlib\\MS_Analog_Status.lvlib\\S0203-MAG-A-R"() -> (w428:dbl)  [unwired: 1 in, 1 out]
    n159 = Multiply(x=w46, y=w45) -> (x*y=w17:dbl)
    n160 = Multiply(x=w44, y=w43) -> (x*y=w16:dbl)
    n161 = Subtract(x=w21, y=w20) -> (x-y=w18:dbl)
    n162 = Multiply(x=w429, y=12.2) -> (x*y=→"Node Voltage":dbl)
    n163 = Subtract(x=w42, y=w39) -> (x-y=w40:dbl)
    n164 = Subtract(x=w27, y=w22) -> (x-y=w26:dbl)
    n165 = Multiply(x=w422, y=12.2) -> (x*y=→"Node Voltage":dbl)
    n166 = Multiply(x=w423, y=12.2) -> (x*y=→"Node Voltage":dbl)
    n167 = Multiply(x=w426, y=12.2) -> (x*y=→"Node Voltage":dbl)
    n168 = Multiply(x=w421, y=12.2) -> (x*y=→"Node Voltage":dbl)
    n169 = Subtract(x=w34, y=w28) -> (x-y=w33:dbl)
    n170 = Subtract(x=w39, y=w34) -> (x-y=w38:dbl)
    n171 = Multiply(x=w425, y=12.2) -> (x*y=→"Node Voltage":dbl)
    n172 = Multiply(x=w424, y=12.2) -> (x*y=→"Node Voltage":dbl)
    n173 = case shown="False" w116 {
      tunnel: [w467 w468] -> _
      frame False {
        w466 = 0.0
        n174 = Merge Signals(w466, w466, w466, w466, w466, w466, w466, w466) -> (w467:dynamicdata)
      }
      frame True {
        n175 = Merge Signals(490.0 ("L2"), 149.0 ("L3"), 440.0 ("L4"), 200.0 ("L5"), 370.0 ("L7"), 351.0 ("L8"), 255.0 ("L9"), 330.0 ("L11")) -> (w468:dynamicdata)
      }
    }
    n176 = Multiply(x=12.2, y=w428) -> (x*y=→"Node Voltage":dbl)
    n177 = Multiply(x=12.2, y=w427) -> (x*y=→"Node Voltage":dbl)
    n178 = Multiply(x=1000.0, y=w40) -> (x*y=→"L2":dbl)
    n179 = Subtract(x=w26, y=w21) -> (x-y=w24:dbl)
    n180 = Subtract(x=w33, y=w32) -> (x-y=w30:dbl)
    n181 = Multiply(x=1000.0, y=w18) -> (x*y=→"L9":dbl)
    n182 = Subtract(x=w38, y=w37) -> (x-y=w35:dbl)
    n183 = shared-variable "MGCC\\MGCC_FntStaMach_Finte State Machine.lvlib\\s_MGCC_FntStaMach_Current_State"() -> (w295:string)  [unwired: 1 in, 1 out]
    n184 = Multiply(x=1000.0, y=w30) -> (x*y=→"L4":dbl)
    n185 = Multiply(x=1000.0, y=w24) -> (x*y=→"L7":dbl)
    n186 = Multiply(x=1000.0, y=w28) -> (x*y=→"L5":dbl)
    n187 = Multiply(x=1000.0, y=w35) -> (x*y=→"L3":dbl)
    n188 = Multiply(x=1000.0, y=w22) -> (x*y=→"L8":dbl)
    n189 = Subtract(x=w17, y=w16) -> (x-y=w14:dbl)
    n190 = shared-variable "MGCC\\DNP3_Master_Station_OpalRT.lvlib\\DNP3_Master_Data_Variables.lvlib\\MS_Analog_Status.lvlib\\S0708-APF"() -> (w183:dbl)  [unwired: 1 in, 1 out]
    n191 = shared-variable "MGCC\\DNP3_Master_Station_OpalRT.lvlib\\DNP3_Master_Data_Variables.lvlib\\MS_Analog_Status.lvlib\\S0709-APF"() -> (w185:dbl)  [unwired: 1 in, 1 out]
    n192 = shared-variable "MGCC\\DNP3_Master_Station_OpalRT.lvlib\\DNP3_Master_Data_Variables.lvlib\\MS_Analog_Status.lvlib\\S0307-APF"() -> (w184:dbl)  [unwired: 1 in, 1 out]
    n193 = Multiply(x=1000.0, y=w14) -> (x*y=→"L11":dbl)
    n194 = shared-variable "MGCC\\DNP3_Master_Station_OpalRT.lvlib\\DNP3_Master_Data_Variables.lvlib\\MS_Analog_Status.lvlib\\S1011-APF"() -> (w404:dbl)  [unwired: 1 in, 1 out]
    n195 = shared-variable "MGCC\\DNP3_Master_Station_OpalRT.lvlib\\DNP3_Master_Data_Variables.lvlib\\MS_Analog_Status.lvlib\\S0708-APF"() -> (w119:dbl)  [unwired: 1 in, 1 out]
    n196 = shared-variable "MGCC\\DNP3_Master_Station_OpalRT.lvlib\\DNP3_Master_Data_Variables.lvlib\\MS_Analog_Status.lvlib\\S0910-APF"() -> (w407:dbl)  [unwired: 1 in, 1 out]
    n197 = shared-variable "MGCC\\DNP3_Master_Station_OpalRT.lvlib\\DNP3_Master_Data_Variables.lvlib\\MS_Analog_Status.lvlib\\S0709-APF"() -> (w408:dbl)  [unwired: 1 in, 1 out]
    n198 = shared-variable "MGCC\\DNP3_Master_Station_OpalRT.lvlib\\DNP3_Master_Data_Variables.lvlib\\MS_Analog_Status.lvlib\\S0304-APF"() -> (w415:dbl)  [unwired: 1 in, 1 out]
    n199 = shared-variable "MGCC\\DNP3_Master_Station_OpalRT.lvlib\\DNP3_Master_Data_Variables.lvlib\\MS_Analog_Status.lvlib\\S1011-APF"() -> (w172:dbl)  [unwired: 1 in, 1 out]
    n200 = shared-variable "MGCC\\DNP3_Master_Station_OpalRT.lvlib\\DNP3_Master_Data_Variables.lvlib\\MS_Analog_Status.lvlib\\S0405-APF"() -> (w414:dbl)  [unwired: 1 in, 1 out]
    n201 = shared-variable "MGCC\\DNP3_Master_Station_OpalRT.lvlib\\DNP3_Master_Data_Variables.lvlib\\MS_Analog_Status.lvlib\\S0405-APF"() -> (w133:dbl)  [unwired: 1 in, 1 out]
    n202 = shared-variable "MGCC\\DNP3_Master_Station_OpalRT.lvlib\\DNP3_Master_Data_Variables.lvlib\\MS_Analog_Status.lvlib\\S0910-APF"() -> (w173:dbl)  [unwired: 1 in, 1 out]
    n203 = shared-variable "BESS LC\\DNP3_Master_Station_OpalRT.lvlib\\DNP3_Master_Data_Variables.lvlib\\MS_Analog_Status.lvlib\\BESS-APO"() -> (w176:dbl)  [unwired: 1 in, 1 out]
    n204 = shared-variable "MGCC\\DNP3_Master_Station_OpalRT.lvlib\\DNP3_Master_Data_Variables.lvlib\\MS_Analog_Status.lvlib\\S0406-APF"() -> (w412:dbl)  [unwired: 1 in, 1 out]
    n205 = shared-variable "MGCC\\DNP3_Master_Station_OpalRT.lvlib\\DNP3_Master_Data_Variables.lvlib\\MS_Analog_Status.lvlib\\S0203-APF"() -> (w193:dbl)  [unwired: 1 in, 1 out]
    n206 = shared-variable "PV LC\\DNP3_Master_Station_Template.lvlib\\DNP3_Master_Data_Variables.lvlib\\MS_Analog_Status.lvlib\\PV-APO"() -> (w175:dbl)  [unwired: 1 in, 1 out]
    n207 = shared-variable "MGCC\\DNP3_Master_Station_OpalRT.lvlib\\DNP3_Master_Data_Variables.lvlib\\MS_Analog_Status.lvlib\\S1114-APF"() -> (w403:dbl)  [unwired: 1 in, 1 out]
    n208 = shared-variable "MGCC\\DNP3_Master_Station_OpalRT.lvlib\\DNP3_Master_Data_Variables.lvlib\\MS_Analog_Status.lvlib\\S0304-APF"() -> (w192:dbl)  [unwired: 1 in, 1 out]
    n209 = shared-variable "MGCC\\DNP3_Master_Station_OpalRT.lvlib\\DNP3_Master_Data_Variables.lvlib\\MS_Analog_Status.lvlib\\S0307-APF"() -> (w194:dbl)  [unwired: 1 in, 1 out]
    n210 = Absolute Value(x=w183) -> (abs(x)=w181:dbl)
    n211 = Absolute Value(x=w184) -> (abs(x)=w182:dbl)
    n212 = shared-variable "MGCC\\DNP3_Master_Station_OpalRT.lvlib\\DNP3_Master_Data_Variables.lvlib\\MS_Analog_Status.lvlib\\S0102-APF"() -> (w420:dbl)  [unwired: 1 in, 1 out]
    n213 = Absolute Value(x=w185) -> (abs(x)=w180:dbl)
    n214 = shared-variable "MGCC\\DNP3_Master_Station_OpalRT.lvlib\\DNP3_Master_Data_Variables.lvlib\\MS_Analog_Status.lvlib\\S0203-APF"() -> (w419:dbl)  [unwired: 1 in, 1 out]
    n215 = case shown="\"State3:GC\"" w295 {
      tunnel: ["Microgrid State: \nOutage" "Microgrid State: \nGrid Connected" "Microgrid State: \nIslanded" "Microgrid State: \nGrid Connected" "Microgrid State: \nGrid Connected" "Microgrid State: \nIslanded" "Microgrid State: \nIslanded" "Current State:\nAbnormal" "Current State:\nFault" "Microgrid State: \nOutage"] -> w88
      tunnel: [w595 w598 w608 w611 w621 w631 w634 w637 w640 w643] -> w91
      tunnel: [u32 16748842 u32 1985280 u32 16711680 u32 1985280 u32 1985280 u32 16711680 u32 16711680 u32 0 u32 0 u32 16748842] -> w89
      frame "State2:STD" {
        n216 = shared-variable "MGCC\\MGCC_PQBal_Internal.lvlib\\MGCC_PQBal_Internal_main.lvlib\\f_MGCC_PQBal_Internal_main_Loadtot_P"() -> (w595:dbl)  [unwired: 1 in, 1 out]
      }
      frame "State3:GC" {
        n217 = shared-variable "PV LC\\DNP3_Master_Station_Template.lvlib\\DNP3_Master_Data_Variables.lvlib\\MS_Analog_Status.lvlib\\PV-APO"() -> (w601:dbl)  [unwired: 1 in, 1 out]
        n218 = shared-variable "MGCC\\DNP3_Master_Station_OpalRT.lvlib\\DNP3_Master_Data_Variables.lvlib\\MS_Analog_Status.lvlib\\S0102-APF"() -> (w605:dbl)  [unwired: 1 in, 1 out]
        n219 = shared-variable "BESS LC\\DNP3_Master_Station_OpalRT.lvlib\\DNP3_Master_Data_Variables.lvlib\\MS_Analog_Status.lvlib\\BESS-APO"() -> (w602:dbl)  [unwired: 1 in, 1 out]
        n220 = shared-variable "MGCC\\DNP3_Master_Station_OpalRT.lvlib\\DNP3_Master_Data_Variables.lvlib\\MS_Analog_Status.lvlib\\S0406-APF"() -> (w604:dbl)  [unwired: 1 in, 1 out]
        n221 = shared-variable "MGCC\\DNP3_Master_Station_OpalRT.lvlib\\DNP3_Master_Data_Variables.lvlib\\MS_Analog_Status.lvlib\\S1114-APF"() -> (w603:dbl)  [unwired: 1 in, 1 out]
        n222 = Compound Arithmetic op=ADD(w605, w604, w603, w602, w601) -> (w599:dbl)
        n223 = Multiply(x=1000.0, y=w599) -> (x*y=w598:dbl)
      }
      frame "State4:ISD" {
        n224 = shared-variable "MGCC\\MGCC_PQBal_Internal.lvlib\\MGCC_PQBal_Internal_main.lvlib\\f_MGCC_PQBal_Internal_main_Loadtot_P"() -> (w608:dbl)  [unwired: 1 in, 1 out]
      }
      frame "State5:G2I_IN" {
        n225 = shared-variable "PV LC\\DNP3_Master_Station_Template.lvlib\\DNP3_Master_Data_Variables.lvlib\\MS_Analog_Status.lvlib\\PV-APO"() -> (w614:dbl)  [unwired: 1 in, 1 out]
        n226 = shared-variable "MGCC\\DNP3_Master_Station_OpalRT.lvlib\\DNP3_Master_Data_Variables.lvlib\\MS_Analog_Status.lvlib\\S0102-APF"() -> (w618:dbl)  [unwired: 1 in, 1 out]
        n227 = shared-variable "BESS LC\\DNP3_Master_Station_OpalRT.lvlib\\DNP3_Master_Data_Variables.lvlib\\MS_Analog_Status.lvlib\\BESS-APO"() -> (w615:dbl)  [unwired: 1 in, 1 out]
        n228 = shared-variable "MGCC\\DNP3_Master_Station_OpalRT.lvlib\\DNP3_Master_Data_Variables.lvlib\\MS_Analog_Status.lvlib\\S0406-APF"() -> (w617:dbl)  [unwired: 1 in, 1 out]
        n229 = shared-variable "MGCC\\DNP3_Master_Station_OpalRT.lvlib\\DNP3_Master_Data_Variables.lvlib\\MS_Analog_Status.lvlib\\S1114-APF"() -> (w616:dbl)  [unwired: 1 in, 1 out]
        n230 = Compound Arithmetic op=ADD(w618, w616, w617, w615, w614) -> (w612:dbl)
        n231 = Multiply(x=1000.0, y=w612) -> (x*y=w611:dbl)
      }
      frame "State6:G2I_UN" {
        n232 = shared-variable "PV LC\\DNP3_Master_Station_Template.lvlib\\DNP3_Master_Data_Variables.lvlib\\MS_Analog_Status.lvlib\\PV-APO"() -> (w624:dbl)  [unwired: 1 in, 1 out]
        n233 = shared-variable "MGCC\\DNP3_Master_Station_OpalRT.lvlib\\DNP3_Master_Data_Variables.lvlib\\MS_Analog_Status.lvlib\\S0102-APF"() -> (w628:dbl)  [unwired: 1 in, 1 out]
        n234 = shared-variable "BESS LC\\DNP3_Master_Station_OpalRT.lvlib\\DNP3_Master_Data_Variables.lvlib\\MS_Analog_Status.lvlib\\BESS-APO"() -> (w625:dbl)  [unwired: 1 in, 1 out]
        n235 = shared-variable "MGCC\\DNP3_Master_Station_OpalRT.lvlib\\DNP3_Master_Data_Variables.lvlib\\MS_Analog_Status.lvlib\\S0406-APF"() -> (w627:dbl)  [unwired: 1 in, 1 out]
        n236 = shared-variable "MGCC\\DNP3_Master_Station_OpalRT.lvlib\\DNP3_Master_Data_Variables.lvlib\\MS_Analog_Status.lvlib\\S1114-APF"() -> (w626:dbl)  [unwired: 1 in, 1 out]
        n237 = Compound Arithmetic op=ADD(w628, w626, w627, w625, w624) -> (w622:dbl)
        n238 = Multiply(x=1000.0, y=w622) -> (x*y=w621:dbl)
      }
      frame "State7:I2G" {
        n239 = shared-variable "MGCC\\MGCC_PQBal_Internal.lvlib\\MGCC_PQBal_Internal_main.lvlib\\f_MGCC_PQBal_Internal_main_Loadtot_P"() -> (w631:dbl)  [unwired: 1 in, 1 out]
      }
      frame "State8:BKS" {
        n240 = shared-variable "MGCC\\MGCC_PQBal_Internal.lvlib\\MGCC_PQBal_Internal_main.lvlib\\f_MGCC_PQBal_Internal_main_Loadtot_P"() -> (w634:dbl)  [unwired: 1 in, 1 out]
      }
      frame "State9:ABN" {
        n241 = shared-variable "MGCC\\MGCC_PQBal_Internal.lvlib\\MGCC_PQBal_Internal_main.lvlib\\f_MGCC_PQBal_Internal_main_Loadtot_P"() -> (w637:dbl)  [unwired: 1 in, 1 out]
      }
      frame "State10:FLT" {
        n242 = shared-variable "MGCC\\MGCC_PQBal_Internal.lvlib\\MGCC_PQBal_Internal_main.lvlib\\f_MGCC_PQBal_Internal_main_Loadtot_P"() -> (w640:dbl)  [unwired: 1 in, 1 out]
      }
      frame "State1:OFF", Default {
        n243 = shared-variable "MGCC\\MGCC_PQBal_Internal.lvlib\\MGCC_PQBal_Internal_main.lvlib\\f_MGCC_PQBal_Internal_main_Loadtot_P"() -> (w643:dbl)  [unwired: 1 in, 1 out]
      }
    }
    "Current State" <- w88
    "Total Load" <- w91
    n244 = Absolute Value(x=w407) -> (abs(x)=w178:dbl)
    n245 = Absolute Value(x=w408) -> (abs(x)=w179:dbl)
    n246 = Absolute Value(x=w173) -> (abs(x)=w171:dbl)
    n247 = Absolute Value(x=w415) -> (abs(x)=w188:dbl)
    n248 = Absolute Value(x=w172) -> (abs(x)=w170:dbl)
    n249 = Absolute Value(x=w414) -> (abs(x)=w187:dbl)
    n250 = Absolute Value(x=w193) -> (abs(x)=w191:dbl)
    n251 = Subtract(x=w179, y=w178) -> (x-y=w406:dbl)
    n252 = Subtract(x=w180, y=w182) -> (x-y=w410:dbl)
    n253 = Subtract(x=w410, y=w181) -> (x-y=w409:dbl)
    n254 = Absolute Value(x=w412) -> (abs(x)=w186:dbl)
    n255 = global write "Global communication output.vi" "Analog output"("test com") -> ()
    n256 = Subtract(x=w188, y=w187) -> (x-y=w413:dbl)
    n257 = Absolute Value(x=w420) -> (abs(x)=w196:dbl)
    n258 = Subtract(x=w404, y=w403) -> (x-y=w402:dbl)
    n259 = Absolute Value(x=w419) -> (abs(x)=w195:dbl)
    n260 = Absolute Value(x=w194) -> (abs(x)=w190:dbl)
    n261 = Absolute Value(x=w192) -> (abs(x)=w189:dbl)
    n262 = Subtract(x=w413, y=w186) -> (x-y=w411:dbl)
    n263 = Add(x=w176, y=w175) -> (x+y=w174:dbl)
    n264 = Subtract(x=w174, y=w171) -> (x-y=w405:dbl)
    n265 = Subtract(x=w405, y=w170) -> (x-y=w177:dbl)
    n266 = Absolute Value(x=w409) -> (abs(x)=w120:dbl)
    n267 = Absolute Value(x=w406) -> (abs(x)=w118:dbl)
    n268 = Subtract(x=w190, y=w191) -> (x-y=w417:dbl)
    n269 = Subtract(x=w196, y=w195) -> (x-y=w418:dbl)
    n270 = Absolute Value(x=w411) -> (abs(x)=w121:dbl)
    n271 = Subtract(x=w417, y=w189) -> (x-y=w416:dbl)
    n272 = Absolute Value(x=w177) -> (abs(x)=w129:dbl)
    n273 = Absolute Value(x=w418) -> (abs(x)=w117:dbl)
    n274 = Absolute Value(x=w402) -> (abs(x)=w115:dbl)
    n275 = Absolute Value(x=w416) -> (abs(x)=w122:dbl)
    n276 = shared-variable "MGCC\\DNP3_Master_Station_OpalRT.lvlib\\DNP3_Master_Data_Variables.lvlib\\MS_Analog_Status.lvlib\\S0910-status"() -> (w78:dbl)  [unwired: 1 in, 1 out]
    n277 = shared-variable "MGCC\\DNP3_Master_Station_OpalRT.lvlib\\DNP3_Master_Data_Variables.lvlib\\MS_Analog_Status.lvlib\\S0910-APF"() -> (w79:dbl)  [unwired: 1 in, 1 out]
    n278 = shared-variable "BESS LC\\DNP3_Master_Station_OpalRT.lvlib\\DNP3_Master_Data_Variables.lvlib\\MS_Analog_Status.lvlib\\BESS-APO"() -> (w71:dbl)  [unwired: 1 in, 1 out]
    n279 = shared-variable "PV LC\\DNP3_Master_Station_Template.lvlib\\DNP3_Master_Data_Variables.lvlib\\MS_Analog_Status.lvlib\\PV-APO"() -> (w70:dbl)  [unwired: 1 in, 1 out]
    n280 = shared-variable "MGCC\\DNP3_Master_Station_OpalRT.lvlib\\DNP3_Master_Data_Variables.lvlib\\MS_Analog_Status.lvlib\\S1011-APF"() -> (w77:dbl)  [unwired: 1 in, 1 out]
    n281 = shared-variable "MGCC\\DNP3_Master_Station_OpalRT.lvlib\\DNP3_Master_Data_Variables.lvlib\\MS_Analog_Status.lvlib\\S1011-status"() -> (w76:dbl)  [unwired: 1 in, 1 out]
    n282 = Multiply(x=1000.0, y=w115) -> ()  [unwired: 1 out]
    n283 = Multiply(x=1000.0, y=w133) -> ()  [unwired: 1 out]
    n284 = Multiply(x=1000.0, y=w122) -> ()  [unwired: 1 out]
    n285 = shared-variable "MGCC\\DNP3_Master_Station_OpalRT.lvlib\\DNP3_Master_Data_Variables.lvlib\\MS_Analog_Status.lvlib\\S0406-FREQ-R"() -> (w400:dbl)  [unwired: 1 in, 1 out]
    n286 = Multiply(x=1000.0, y=w120) -> ()  [unwired: 1 out]
    n287 = Multiply(x=1000.0, y=w129) -> ()  [unwired: 1 out]
    n288 = Multiply(x=w79, y=w78) -> (x*y=w73:dbl)
    n289 = Multiply(x=w77, y=w76) -> (x*y=w75:dbl)
    n290 = Multiply(x=1000.0, y=w121) -> ()  [unwired: 1 out]
    n291 = shared-variable "MGCC\\DNP3_Master_Station_OpalRT.lvlib\\DNP3_Master_Data_Variables.lvlib\\MS_Analog_Status.lvlib\\S0406-ANG-DIFF"() -> (w150:dbl)  [unwired: 1 in, 1 out]
    n292 = shared-variable "MGCC\\DNP3_Master_Station_OpalRT.lvlib\\DNP3_Master_Data_Variables.lvlib\\MS_Analog_Status.lvlib\\S0910-ANG-DIFF"() -> (w147:dbl)  [unwired: 1 in, 1 out]
    n293 = shared-variable "MGCC\\DNP3_Master_Station_OpalRT.lvlib\\DNP3_Master_Data_Variables.lvlib\\MS_Analog_Status.lvlib\\S1114-ANG-DIFF"() -> (w144:dbl)  [unwired: 1 in, 1 out]
    n294 = shared-variable "MGCC\\DNP3_Master_Station_OpalRT.lvlib\\DNP3_Master_Data_Variables.lvlib\\MS_Analog_Status.lvlib\\S0102-FREQ-L"() -> (w401:dbl)  [unwired: 1 in, 1 out]
    n295 = Multiply(x=1000.0, y=w119) -> ()  [unwired: 1 out]
    n296 = Multiply(x=1000.0, y=w117) -> ()  [unwired: 1 out]
    n297 = Multiply(x=1000.0, y=w118) -> ()  [unwired: 1 out]
    n298 = shared-variable "MGCC\\DNP3_Master_Station_OpalRT.lvlib\\DNP3_Master_Data_Variables.lvlib\\MS_Analog_Status.lvlib\\S0203-ANG-DIFF"() -> (w153:dbl)  [unwired: 1 in, 1 out]
    n299 = Multiply(x=w75, y=-1.0) -> (x*y=w72:dbl)
    n300 = control-ref of="Current State"() -> (w90:refnum<vi>)
    n301 = shared-variable "MGCC\\DNP3_Master_Station_OpalRT.lvlib\\DNP3_Master_Data_Variables.lvlib\\MS_Analog_Status.lvlib\\S1114-FREQ-R"() -> (w399:dbl)  [unwired: 1 in, 1 out]
    n302 = shared-variable "MGCC\\DNP3_Master_Station_OpalRT.lvlib\\DNP3_Master_Data_Variables.lvlib\\MS_Analog_Status.lvlib\\S1011-ANG-DIFF"() -> (w141:dbl)  [unwired: 1 in, 1 out]
    n303 = shared-variable "PV LC\\DNP3_Master_Station_Template.lvlib\\DNP3_Master_Data_Variables.lvlib\\MS_Analog_Status.lvlib\\PV-APO"() -> (w294:dbl)  [unwired: 1 in, 1 out]
    n304 = shared-variable "PV LC\\DNP3_Master_Station_Template.lvlib\\DNP3_Master_Data_Variables.lvlib\\MS_Analog_Status.lvlib\\PV-APO"() -> (w392:dbl)  [unwired: 1 in, 1 out]
    n305 = shared-variable "MGCC\\DNP3_Master_Station_OpalRT.lvlib\\DNP3_Master_Data_Variables.lvlib\\MS_Analog_Status.lvlib\\S0102-APF"() -> (w396:dbl)  [unwired: 1 in, 1 out]
    n306 = shared-variable "BESS LC\\DNP3_Master_Station_OpalRT.lvlib\\DNP3_Master_Data_Variables.lvlib\\MS_Analog_Status.lvlib\\BESS-APO"() -> (w393:dbl)  [unwired: 1 in, 1 out]
    n307 = shared-variable "BESS LC\\DNP3_Master_Station_OpalRT.lvlib\\DNP3_Master_Data_Variables.lvlib\\MS_Analog_Status.lvlib\\BESS-FREQ"() -> (w398:dbl)  [unwired: 1 in, 1 out]
    n308 = shared-variable "MGCC\\MGCC_PVFcst_dataIO.lvlib\\f_MGCC_PVFcst_FcstPV"() -> (→"PV Forecast":dbl[])  [unwired: 1 in, 1 out]
    n309 = shared-variable "MGCC\\DNP3_Master_Station_OpalRT.lvlib\\DNP3_Master_Data_Variables.lvlib\\MS_Analog_Status.lvlib\\S0406-APF"() -> (w395:dbl)  [unwired: 1 in, 1 out]
    n310 = shared-variable "MGCC\\DNP3_Master_Station_OpalRT.lvlib\\DNP3_Master_Data_Variables.lvlib\\MS_Analog_Status.lvlib\\S1114-APF"() -> (w394:dbl)  [unwired: 1 in, 1 out]
    n311 = property on="Property Node" class="Str"(reference=w90, "Text.FontColor"=w89) -> ()  [unwired: 1 in, 2 out]
    n312 = Compound Arithmetic op=ADD(w71, w70, w73, w72) -> (w68:dbl)
    n313 = Multiply(x=w294, y=1000.0) -> (x*y=→"PV Output" →"Max PV":dbl)
    n314 = shared-variable "MGCC\\MGCC_FntStaMach_Finte State Machine.lvlib\\b_MGCC_FntStaMach_reset"("RESET") -> ()  [unwired: 1 in, 1 out]
    n315 = Bundle("Double"=w401, "Double"=w400, "Double"=w399, "Double"=w398) -> (→"Frequency":T2)  [unwired: 1 in]
    n316 = Multiply(x=57.3, y=w147) -> (x*y=→"Angle Diff.\n09-10":dbl)
    n317 = Multiply(x=1000.0, y=w68) -> (x*y=→"L10":dbl)
    n318 = case shown="\"Cloudy Day\"" "Irradiance" {
      tunnel: [1 2 0] -> w96
      frame "Sunny Day" {
      }
      frame "Cloudy Day" {
      }
      frame "Manually Control", Default {
      }
    }
    n319 = case shown="True" "RESET" {
      frame False {
      }
      frame True {
        w591 = FALSE ("S0102-status-ctrl")
        w593 = 0.0
        n320 = shared-variable ".\\DNP3_Master_Station_OpalRT.lvlib\\DNP3_Master_Data_Variables.lvlib\\MS_Analog_Control.lvlib\\S0203-STATUS-CTRL"(w593) -> ()  [unwired: 1 in, 1 out]
        n321 = shared-variable ".\\DNP3_Master_Station_OpalRT.lvlib\\DNP3_Master_Data_Variables.lvlib\\MS_Analog_Control.lvlib\\S0304-STATUS-CTRL"(w593) -> ()  [unwired: 1 in, 1 out]
        n322 = shared-variable ".\\DNP3_Master_Station_OpalRT.lvlib\\DNP3_Master_Data_Variables.lvlib\\MS_Analog_Control.lvlib\\S0307-STATUS-CTRL"(w593) -> ()  [unwired: 1 in, 1 out]
        n323 = shared-variable ".\\DNP3_Master_Station_OpalRT.lvlib\\DNP3_Master_Data_Variables.lvlib\\MS_Analog_Control.lvlib\\S0405-STATUS-CTRL"(w593) -> ()  [unwired: 1 in, 1 out]
        n324 = shared-variable "MGCC\\MGCC_FntStaMach_Finte State Machine.lvlib\\s_MGCC_FntStaMach_Current_State"("State2:STD" ("s_MGCC_FntStaMach_Current_State")) -> ()  [unwired: 1 in, 1 out]
        n325 = shared-variable "MGCC\\MGCC_BlkStart_Output.lvlib\\b_MGCC_BlkStart_Output_success_flag"(w591) -> ()  [unwired: 1 in, 1 out]
        n326 = shared-variable "MGCC\\DNP3_Master_Station_OpalRT.lvlib\\DNP3_Master_Data_Variables.lvlib\\MS_Binary_Control.lvlib\\S0102-status-ctrl"(w591) -> ()  [unwired: 1 in, 1 out]
        n327 = shared-variable "MGCC\\MGCC_PQBal_Internal.lvlib\\b_MGCC_PQBal_output_flag"(w591) -> ()  [unwired: 1 in, 1 out]
        n328 = shared-variable ".\\DNP3_Master_Station_OpalRT.lvlib\\DNP3_Master_Data_Variables.lvlib\\MS_Analog_Control.lvlib\\S0708-STATUS-CTRL"(w593) -> ()  [unwired: 1 in, 1 out]
        n329 = shared-variable ".\\DNP3_Master_Station_OpalRT.lvlib\\DNP3_Master_Data_Variables.lvlib\\MS_Analog_Control.lvlib\\S0910-STATUS-CTRL"(w593) -> ()  [unwired: 1 in, 1 out]
        n330 = shared-variable ".\\DNP3_Master_Station_OpalRT.lvlib\\DNP3_Master_Data_Variables.lvlib\\MS_Analog_Control.lvlib\\S1011-STATUS-CTRL"(w593) -> ()  [unwired: 1 in, 1 out]
        n331 = shared-variable "MGCC\\MGCC_BlkStart_Output.lvlib\\b_MGCC_BlkStart_Output_failure_flag5"(w591) -> ()  [unwired: 1 in, 1 out]
        n332 = shared-variable ".\\DNP3_Master_Station_OpalRT.lvlib\\DNP3_Master_Data_Variables.lvlib\\MS_Analog_Control.lvlib\\S0709-STATUS-CTRL"(w593) -> ()  [unwired: 1 in, 1 out]
        n333 = shared-variable ".\\DNP3_Master_Station_OpalRT.lvlib\\DNP3_Master_Data_Variables.lvlib\\MS_Analog_Control.lvlib\\S0406-STATUS-CTRL"(w593) -> ()  [unwired: 1 in, 1 out]
        n334 = shared-variable ".\\DNP3_Master_Station_OpalRT.lvlib\\DNP3_Master_Data_Variables.lvlib\\MS_Analog_Control.lvlib\\S0102-STATUS-CTRL"(w593) -> ()  [unwired: 1 in, 1 out]
        n335 = shared-variable ".\\DNP3_Master_Station_OpalRT.lvlib\\DNP3_Master_Data_Variables.lvlib\\MS_Analog_Control.lvlib\\S1114-STATUS-CTRL"(w593) -> ()  [unwired: 1 in, 1 out]
        n336 = shared-variable "PV LC\\DNP3_Master_Station_Template.lvlib\\DNP3_Master_Data_Variables.lvlib\\MS_Analog_Control.lvlib\\PV-STATUS-CTRL"(w593) -> ()  [unwired: 1 in, 1 out]
        n337 = shared-variable "BESS LC\\DNP3_Master_Station_OpalRT.lvlib\\DNP3_Master_Data_Variables.lvlib\\MS_Analog_Control.lvlib\\BESS-STATUS-CTRL"(w593) -> ()  [unwired: 1 in, 1 out]
      }
    }
    n338 = shared-variable "BESS LC\\DNP3_Master_Station_OpalRT.lvlib\\DNP3_Master_Data_Variables.lvlib\\MS_Analog_Status.lvlib\\BESS-STATUS"() -> (w358:dbl)  [unwired: 1 in, 1 out]
    n339 = shared-variable "MGCC\\DNP3_Master_Station_OpalRT.lvlib\\DNP3_Master_Data_Variables.lvlib\\MS_Analog_Status.lvlib\\S1011-status"() -> (w363:dbl)  [unwired: 1 in, 1 out]
    n340 = shared-variable "PV LC\\DNP3_Master_Station_Template.lvlib\\DNP3_Master_Data_Variables.lvlib\\MS_Analog_Status.lvlib\\PV-STATUS"() -> (w360:dbl)  [unwired: 1 in, 1 out]
    n341 = Multiply(x=57.3, y=w141) -> (x*y=→"Angle Diff.\n10-11":dbl)
    n342 = shared-variable "MGCC\\DNP3_Master_Station_OpalRT.lvlib\\DNP3_Master_Data_Variables.lvlib\\MS_Analog_Status.lvlib\\S0910-status"() -> (w365:dbl)  [unwired: 1 in, 1 out]
    n343 = Multiply(x=57.3, y=w144) -> (x*y=→"Angle Diff.\n11-14":dbl)
    n344 = shared-variable "MGCC\\DNP3_Master_Station_OpalRT.lvlib\\DNP3_Master_Data_Variables.lvlib\\MS_Analog_Status.lvlib\\S0709-status"() -> (w371:dbl)  [unwired: 1 in, 1 out]
    n345 = shared-variable "MGCC\\DNP3_Master_Station_OpalRT.lvlib\\DNP3_Master_Data_Variables.lvlib\\MS_Analog_Status.lvlib\\S0708-status"() -> (w372:dbl)  [unwired: 1 in, 1 out]
    n346 = shared-variable "MGCC\\MGCC_FntStaMach_Finte State Machine.lvlib\\b_MGCC_FntStaMach_All_Loop_Stop"("Stop") -> ()  [unwired: 1 in, 1 out]
    n347 = Multiply(x=57.3, y=w150) -> (x*y=→"Angle Diff.\n04-06":dbl)
    n348 = shared-variable "MGCC\\DNP3_Master_Station_OpalRT.lvlib\\DNP3_Master_Data_Variables.lvlib\\MS_Analog_Status.lvlib\\S0304-status"() -> (w383:dbl)  [unwired: 1 in, 1 out]
    n349 = shared-variable "MGCC\\DNP3_Master_Station_OpalRT.lvlib\\DNP3_Master_Data_Variables.lvlib\\MS_Analog_Status.lvlib\\S1114-status"() -> (w361:dbl)  [unwired: 1 in, 1 out]
    n350 = Multiply(x=57.3, y=w153) -> (x*y=→"Angle Diff.\n 02-03":dbl)
    n351 = shared-variable "MGCC\\DNP3_Master_Station_OpalRT.lvlib\\DNP3_Master_Data_Variables.lvlib\\MS_Analog_Status.lvlib\\S0405-status"() -> (w376:dbl)  [unwired: 1 in, 1 out]
    n352 = shared-variable "MGCC\\DNP3_Master_Station_OpalRT.lvlib\\DNP3_Master_Data_Variables.lvlib\\MS_Analog_Status.lvlib\\S0406-status"() -> (w373:dbl)  [unwired: 1 in, 1 out]
    n353 = shared-variable "MGCC\\DNP3_Master_Station_OpalRT.lvlib\\DNP3_Master_Data_Variables.lvlib\\MS_Analog_Status.lvlib\\S0307-status"() -> (w375:dbl)  [unwired: 1 in, 1 out]
    n354 = Bundle("Double"=w396, "Double"=w395, "Double"=w394, "Double"=w393, "Double"=w392) -> (→"Sources Power":T1)  [unwired: 1 in]
    n355 = shared-variable "MGCC\\DNP3_Master_Station_OpalRT.lvlib\\DNP3_Master_Data_Variables.lvlib\\MS_Analog_Status.lvlib\\S0203-status"() -> (w385:dbl)  [unwired: 1 in, 1 out]
    n356 = shared-variable "MGCC\\DNP3_Master_Station_OpalRT.lvlib\\DNP3_Master_Data_Variables.lvlib\\MS_Analog_Status.lvlib\\S0102-status"() -> (w389:dbl)  [unwired: 1 in, 1 out]
    n357 = shared-variable "PV LC\\DNP3_Master_Station_Template.lvlib\\DNP3_Master_Data_Variables.lvlib\\MS_Analog_Control.lvlib\\PV-RESERVED4"(w96) -> ()  [unwired: 1 in, 1 out]
    n358 = shared-variable "BESS LC\\DNP3_Master_Station_OpalRT.lvlib\\DNP3_Master_Data_Variables.lvlib\\MS_Analog_Status.lvlib\\BESS-STATUS"() -> (w352:dbl)  [unwired: 1 in, 1 out]
    n359 = shared-variable "PV LC\\DNP3_Master_Station_Template.lvlib\\DNP3_Master_Data_Variables.lvlib\\MS_Analog_Status.lvlib\\PV-STATUS"() -> (w353:dbl)  [unwired: 1 in, 1 out]
    n360 = Greater?(x=w371, y=0.5) -> (0:→"S0709":bool)
    n361 = Greater?(x=w365, y=0.5) -> (0:→"S0910":bool)
    n362 = Greater?(x=w363, y=0.5) -> (0:→"S1011":bool)
    n363 = Greater?(x=w389, y=0.5) -> (0:→"S0102" →"G1":bool)
    n364 = Greater?(x=w372, y=0.5) -> (0:→"S0708":bool)
    n365 = Greater?(x=w385, y=0.5) -> (0:→"S0203":bool)
    n366 = Greater?(x=w360, y=0.5) -> (0:→"S1012":bool)
    n367 = Greater?(x=w358, y=0.5) -> (0:→"W11" →"S1013":bool)
    n368 = shared-variable "MGCC\\DNP3_Master_Station_OpalRT.lvlib\\DNP3_Master_Data_Variables.lvlib\\MS_Analog_Status.lvlib\\S0102-ANG-DIFF"() -> (w169:dbl)  [unwired: 1 in, 1 out]
    n369 = Greater?(x=w383, y=0.5) -> (0:→"S0304":bool)
    n370 = Greater?(x=w376, y=0.5) -> (0:→"S0405":bool)
    n371 = Greater?(x=w375, y=0.5) -> (0:→"S0307":bool)
    n372 = Greater?(x=w373, y=0.5) -> (0:→"S0406" →"G6":bool)
    n373 = Greater?(x=w361, y=0.5) -> (0:→"S1114" →"G14":bool)
    n374 = shared-variable "MGCC\\DNP3_Master_Station_OpalRT.lvlib\\DNP3_Master_Data_Variables.lvlib\\MS_Analog_Status.lvlib\\S0307-ANG-DIFF"() -> (w162:dbl)  [unwired: 1 in, 1 out]
    n375 = shared-variable "MGCC\\DNP3_Master_Station_OpalRT.lvlib\\DNP3_Master_Data_Variables.lvlib\\MS_Analog_Status.lvlib\\S0709-ANG-DIFF"() -> (w165:dbl)  [unwired: 1 in, 1 out]
    n376 = shared-variable "MGCC\\DNP3_Master_Station_OpalRT.lvlib\\DNP3_Master_Data_Variables.lvlib\\MS_Analog_Status.lvlib\\S0405-ANG-DIFF"() -> (w155:dbl)  [unwired: 1 in, 1 out]
    n377 = shared-variable "BESS LC\\DNP3_Master_Station_OpalRT.lvlib\\DNP3_Master_Data_Variables.lvlib\\MS_Analog_Status.lvlib\\BESS-APO"() -> (w297:dbl)  [unwired: 1 in, 1 out]
    n378 = shared-variable "MGCC\\MGCC_FntStaMach_Functions.lvlib\\b_MGCC_FntStaMach_state_estimation_enable"() -> (→"State Estimation":bool)  [unwired: 1 in, 1 out]
    n379 = shared-variable "MGCC\\DNP3_Master_Station_OpalRT.lvlib\\DNP3_Master_Data_Variables.lvlib\\MS_Analog_Status.lvlib\\S0304-ANG-DIFF"() -> (w159:dbl)  [unwired: 1 in, 1 out]
    n380 = shared-variable "MGCC\\MGCC_OnliTopoIden.lvlib\\f_MGCC_OnliTopoIden_EnergizedMatrix"() -> (w234:dbl[])  [unwired: 1 in, 1 out]
    n381 = Greater?(x=w353, y=0.5) -> (0:w351:bool)
    n382 = Greater?(x=w352, y=0.5) -> (0:w350:bool)
    n383 = Or(x=w351, y=w350) -> ()  [unwired: 1 out]
    n384 = shared-variable "MGCC\\MGCC_EnergyMgmt_dataIO.lvlib\\b_MGCC_EnergyMgmt_Enable"() -> (→"Energy Mgmt.":bool)  [unwired: 1 in, 1 out]
    n385 = shared-variable "BESS LC\\DNP3_Master_Station_OpalRT.lvlib\\DNP3_Master_Data_Variables.lvlib\\MS_Analog_Status.lvlib\\BESS-MAG"() -> ()  [unwired: 1 in, 2 out]
    n386 = shared-variable "MGCC\\MGCC_Commun_mainlib.lvlib\\b_MGCC_Commun_enable"() -> (→"Communication":bool)  [unwired: 1 in, 1 out]
    n387 = shared-variable "BESS LC\\DNP3_Master_Station_OpalRT.lvlib\\DNP3_Master_Data_Variables.lvlib\\MS_Analog_Status.lvlib\\BESS-SOC"() -> (w446:dbl)  [unwired: 1 in, 1 out]
    n388 = shared-variable "MGCC\\MGCC_LoadFcst_dataIO.lvlib\\b_MGCC_LoadFcst_Enable"() -> (→"Load Forecasting":bool)  [unwired: 1 in, 1 out]
    n389 = shared-variable "MGCC\\MGCC.lvlib\\b_MGCC_DataLog_enable"() -> (→"Data Logging":bool)  [unwired: 1 in, 1 out]
    n390 = shared-variable "MGCC\\MGCC_MdlMgmt.lvlib\\b_MGCC_MdlMgmt_done"() -> (→"Topology Identification":bool)  [unwired: 1 in, 1 out]
    n391 = shared-variable "MGCC\\MGCC_BlkStart_Input.lvlib\\b_MGCC_BlkStart_Enable"() -> (→"Black Start":bool)  [unwired: 1 in, 1 out]
    n392 = shared-variable "MGCC\\MGCC_PVFcst_dataIO.lvlib\\b_MGCC_PVFcst_Enable"() -> (→"PV Forecasting":bool)  [unwired: 1 in, 1 out]
    n393 = shared-variable "MGCC\\MGCC_PQBal_Input.lvlib\\b_MGCC_PQBal_enable"() -> (→"PQ Balance":bool)  [unwired: 1 in, 1 out]
    n394 = Multiply(x=57.3, y=w169) -> (x*y=→"Angle Diff.\n01-02":dbl)
    n395 = Multiply(x=57.3, y=w155) -> (x*y=→"Angle Diff.\n04-05":dbl)
    n396 = Multiply(x=57.3, y=w165) -> (x*y=→"Angle Diff.\n07-09":dbl)
    n397 = Multiply(x=57.3, y=w162) -> (x*y=→"Angle Diff.\n03-07":dbl)
    n398 = shared-variable "MGCC\\MGCC_FntStaMach_Finte State Machine.lvlib\\s_MGCC_FntStaMach_Current_State"() -> (w242:string)  [unwired: 1 in, 1 out]
    n399 = Multiply(x=1000.0, y=w297) -> (x*y=→"Battery Output":dbl)
    n400 = Multiply(x=w446, y=100.0) -> (x*y=→"Battery SOC" →"SOC Tank":dbl)
    n401 = Multiply(x=57.3, y=w159) -> (x*y=→"Angle Diff.\n03-04":dbl)
    n402 = Index Array(array=w234, index #1=1 ("index"), index #2=2 ("index"), index #3=3 ("index"), index #4=4 ("index"), index #5=6 ("index"), index #6=7 ("index"), index #7=8 ("index"), index #8=9 ("index"), index #9=10 ("index")) -> (element #1=w231:dbl, element #2=w228:dbl, element #3=w225:dbl, element #4=w222:dbl, element #5=w219:dbl, element #6=w211:dbl, element #7=w206:dbl, element #8=w203:dbl, element #9=w199:dbl)
    n403 = case shown="\"State3:GC\"" w242 {
      tunnel: [w482 w492 w502 w512 w522 w535 w547 w554 w564 w574] -> w241
      tunnel: [w477 w488 w498 w507 w517 w527 w537 w549 w559 w569] -> w238
      frame "State2:STD" {
        n404 = Merge Signals(TRUE ("Resynchronization"), FALSE ("Resynchronization"), FALSE ("Resynchronization"), FALSE ("Resynchronization")) -> (w477:dynamicdata)
        n405 = Merge Signals(TRUE ("Resynchronization"), FALSE ("Resynchronization"), FALSE ("Resynchronization"), FALSE ("Resynchronization")) -> (w482:dynamicdata)
      }
      frame "State3:GC" {
        n406 = Merge Signals(TRUE ("Resynchronization"), FALSE ("Resynchronization"), TRUE ("Resynchronization"), TRUE ("Resynchronization")) -> (w488:dynamicdata)
        n407 = Merge Signals(TRUE ("Resynchronization"), FALSE ("Resynchronization"), TRUE ("Resynchronization"), TRUE ("Resynchronization")) -> (w492:dynamicdata)
      }
      frame "State4:ISD" {
        n408 = Merge Signals(TRUE ("Resynchronization"), FALSE ("Resynchronization"), TRUE ("Resynchronization"), TRUE ("Resynchronization")) -> (w498:dynamicdata)
        n409 = Merge Signals(TRUE ("Resynchronization"), FALSE ("Resynchronization"), TRUE ("Resynchronization"), TRUE ("Resynchronization")) -> (w502:dynamicdata)
      }
      frame "State5:G2I_IN" {
        n410 = Merge Signals(TRUE ("Resynchronization"), FALSE ("Resynchronization"), TRUE ("Resynchronization"), TRUE ("Resynchronization")) -> (w507:dynamicdata)
        n411 = Merge Signals(TRUE ("Resynchronization"), FALSE ("Resynchronization"), TRUE ("Resynchronization"), TRUE ("Resynchronization")) -> (w512:dynamicdata)
      }
      frame "State6:G2I_UN" {
        n412 = Merge Signals(TRUE ("Resynchronization"), FALSE ("Resynchronization"), TRUE ("Resynchronization"), TRUE ("Resynchronization")) -> (w517:dynamicdata)
        n413 = Merge Signals(TRUE ("Resynchronization"), FALSE ("Resynchronization"), TRUE ("Resynchronization"), TRUE ("Resynchronization")) -> (w522:dynamicdata)
      }
      frame "State7:I2G" {
        n414 = Merge Signals(TRUE ("Resynchronization"), TRUE ("Resynchronization"), TRUE ("Resynchronization"), TRUE ("Resynchronization")) -> (w535:dynamicdata)
        n415 = Merge Signals(TRUE ("Resynchronization"), TRUE ("Resynchronization"), TRUE ("Resynchronization"), TRUE ("Resynchronization")) -> (w527:dynamicdata)
      }
      frame "State8:BKS" {
        n416 = shared-variable "PV LC\\DNP3_Master_Station_Template.lvlib\\DNP3_Master_Data_Variables.lvlib\\MS_Analog_Status.lvlib\\PV-STATUS"() -> (w546:dbl)  [unwired: 1 in, 1 out]
        n417 = shared-variable "BESS LC\\DNP3_Master_Station_OpalRT.lvlib\\DNP3_Master_Data_Variables.lvlib\\MS_Analog_Status.lvlib\\BESS-STATUS"() -> (w541:dbl)  [unwired: 1 in, 1 out]
        n418 = Greater?(x=w546, y=0.5) -> (0:w544:bool)
        n419 = Merge Signals(TRUE ("Resynchronization"), FALSE ("Resynchronization"), w544, w544) -> (w547:dynamicdata)
        n420 = Greater?(x=w541, y=0.5) -> (0:w539:bool)
        n421 = Merge Signals(TRUE ("Resynchronization"), FALSE ("Resynchronization"), w539, w539) -> (w537:dynamicdata)
      }
      frame "State9:ABN" {
        n422 = Merge Signals(FALSE ("Resynchronization"), FALSE ("Resynchronization"), FALSE ("Resynchronization"), FALSE ("Resynchronization")) -> (w549:dynamicdata)
        n423 = Merge Signals(FALSE ("Resynchronization"), FALSE ("Resynchronization"), FALSE ("Resynchronization"), FALSE ("Resynchronization")) -> (w554:dynamicdata)
      }
      frame "State10:FLT" {
        n424 = Merge Signals(FALSE ("Resynchronization"), FALSE ("Resynchronization"), FALSE ("Resynchronization"), FALSE ("Resynchronization")) -> (w564:dynamicdata)
        n425 = Merge Signals(FALSE ("Resynchronization"), FALSE ("Resynchronization"), FALSE ("Resynchronization"), FALSE ("Resynchronization")) -> (w559:dynamicdata)
      }
      frame "State1:OFF", Default {
        n426 = Merge Signals(FALSE ("Resynchronization"), FALSE ("Resynchronization"), FALSE ("Resynchronization"), FALSE ("Resynchronization")) -> (w569:dynamicdata)
        n427 = Merge Signals(FALSE ("Resynchronization"), FALSE ("Resynchronization"), FALSE ("Resynchronization"), FALSE ("Resynchronization")) -> (w574:dynamicdata)
      }
    }
    n428 = Greater?(x=w231, y=0.5) -> (0:→"W2" →"L2":bool)
    n429 = Greater?(x=w225, y=0.5) -> (0:→"W4" →"L4":bool)
    n430 = Greater?(x=w222, y=0.5) -> (0:→"W6" →"L5":bool)
    n431 = Greater?(x=w228, y=0.5) -> (0:→"W3" →"L3":bool)
    n432 = Greater?(x=w203, y=0.5) -> (0:→"L10" →"W9":bool)
    n433 = Greater?(x=w199, y=0.5) -> (0:→"W12" →"L11":bool)
    n434 = Greater?(x=w211, y=0.5) -> (0:→"L8":bool)
    n435 = Greater?(x=w219, y=0.5) -> (0:→"W7" →"L7":bool)
    n436 = Greater?(x=w206, y=0.5) -> (0:→"L9" →"W8":bool)
    n437 = global write "Global communication output.vi" "Matrix output"("Matrix output") -> ()
    n438 = Split Signals(w238) -> (→"BESS LC" →"Communication":dynamicdata, →"Resynchronization" →"Resynchronization":dynamicdata, →"Active power control":dynamicdata, →"Reactive power control":dynamicdata)  [unwired: 4 in]
    n439 = Split Signals(w241) -> (→"PV LC" →"Communication":dynamicdata, →"Active power control":dynamicdata, →"Reactive power control":dynamicdata)  [unwired: 4 in, 1 out]
    n440 = shared-variable "MGCC\\MGCC_FntStaMach_Finte State Machine.lvlib\\b_MGCC_FntStaMach_All_Loop_Stop"() -> (w2:bool)  [unwired: 1 in, 1 out]
  }
